vi "数字量输入配置.vi"() -> ()   [LabVIEW 2010]
panel:
  in  "数组":u16[](array[numeric]) format="%x"
  in  "保持输入":bool
  out "同步_A2":i32
  out "同步_A1":i32
  in  "数组_输入值":enum16{"0", "1"}[][](array[ring])
  in  "数组_选择?":bool[][](array[boolean])
  in  "btn_置1_5":bool
  in  "btn_置1_4":bool
  in  "btn_置1_3":bool
  in  "btn_置1_2":bool
  in  "btn_全选_5":bool
  in  "btn_全选_4":bool
  in  "btn_全选_3":bool
  in  "btn_全选_2":bool
  in  "btn_置1_1":bool
  in  "btn_全选_1":bool
  in  "CAN端口":u16
  out "light_80":bool
  out "light_79":bool
  out "light_78":bool
  out "light_77":bool
  out "light_76":bool
  out "light_75":bool
  out "light_74":bool
  out "light_73":bool
  out "light_72":bool
  out "light_71":bool
  out "light_70":bool
  out "light_69":bool
  out "light_68":bool
  out "light_67":bool
  out "light_66":bool
  out "light_65":bool
  in  "输入值_73":enum16{"0", "1"}(ring)
  in  "输入值_80":enum16{"0", "1"}(ring)
  in  "输入值_79":enum16{"0", "1"}(ring)
  in  "输入值_78":enum16{"0", "1"}(ring)
  in  "输入值_77":enum16{"0", "1"}(ring)
  in  "输入值_76":enum16{"0", "1"}(ring)
  in  "输入值_75":enum16{"0", "1"}(ring)
  in  "输入值_74":enum16{"0", "1"}(ring)
  in  "输入值_65":enum16{"0", "1"}(ring)
  in  "输入值_72":enum16{"0", "1"}(ring)
  in  "输入值_71":enum16{"0", "1"}(ring)
  in  "输入值_70":enum16{"0", "1"}(ring)
  in  "输入值_69":enum16{"0", "1"}(ring)
  in  "输入值_68":enum16{"0", "1"}(ring)
  in  "输入值_67":enum16{"0", "1"}(ring)
  in  "输入值_66":enum16{"0", "1"}(ring)
  in  "单选_第73路":bool
  in  "单选_第80路":bool
  in  "单选_第79路":bool
  in  "单选_第78路":bool
  in  "单选_第77路":bool
  in  "单选_第76路":bool
  in  "单选_第75路":bool
  in  "单选_第74路":bool
  in  "单选_第65路":bool
  in  "单选_第72路":bool
  in  "单选_第71路":bool
  in  "单选_第70路":bool
  in  "单选_第69路":bool
  in  "单选_第68路":bool
  in  "单选_第67路":bool
  in  "单选_第66路":bool
  out "light_64":bool
  out "light_63":bool
  out "light_62":bool
  out "light_61":bool
  out "light_60":bool
  out "light_59":bool
  out "light_58":bool
  out "light_57":bool
  out "light_56":bool
  out "light_55":bool
  out "light_54":bool
  out "light_53":bool
  out "light_52":bool
  out "light_51":bool
  out "light_50":bool
  out "light_49":bool
  in  "输入值_57":enum16{"0", "1"}(ring)
  in  "输入值_64":enum16{"0", "1"}(ring)
  in  "输入值_63":enum16{"0", "1"}(ring)
  in  "输入值_62":enum16{"0", "1"}(ring)
  in  "输入值_61":enum16{"0", "1"}(ring)
  in  "输入值_60":enum16{"0", "1"}(ring)
  in  "输入值_59":enum16{"0", "1"}(ring)
  in  "输入值_58":enum16{"0", "1"}(ring)
  in  "输入值_49":enum16{"0", "1"}(ring)
  in  "输入值_56":enum16{"0", "1"}(ring)
  in  "输入值_55":enum16{"0", "1"}(ring)
  in  "输入值_54":enum16{"0", "1"}(ring)
  in  "输入值_53":enum16{"0", "1"}(ring)
  in  "输入值_52":enum16{"0", "1"}(ring)
  in  "输入值_51":enum16{"0", "1"}(ring)
  in  "输入值_50":enum16{"0", "1"}(ring)
  in  "单选_第57路":bool
  in  "单选_第64路":bool
  in  "单选_第63路":bool
  in  "单选_第62路":bool
  in  "单选_第61路":bool
  in  "单选_第60路":bool
  in  "单选_第59路":bool
  in  "单选_第58路":bool
  in  "单选_第49路":bool
  in  "单选_第56路":bool
  in  "单选_第55路":bool
  in  "单选_第54路":bool
  in  "单选_第53路":bool
  in  "单选_第52路":bool
  in  "单选_第51路":bool
  in  "单选_第50路":bool
  out "light_48":bool
  out "light_47":bool
  out "light_46":bool
  out "light_45":bool
  out "light_44":bool
  out "light_43":bool
  out "light_42":bool
  out "light_41":bool
  out "light_40":bool
  out "light_39":bool
  out "light_38":bool
  out "light_37":bool
  out "light_36":bool
  out "light_35":bool
  out "light_34":bool
  out "light_33":bool
  in  "输入值_41":enum16{"0", "1"}(ring)
  in  "输入值_48":enum16{"0", "1"}(ring)
  in  "输入值_47":enum16{"0", "1"}(ring)
  in  "输入值_46":enum16{"0", "1"}(ring)
  in  "输入值_45":enum16{"0", "1"}(ring)
  in  "输入值_44":enum16{"0", "1"}(ring)
  in  "输入值_43":enum16{"0", "1"}(ring)
  in  "输入值_42":enum16{"0", "1"}(ring)
  in  "输入值_33":enum16{"0", "1"}(ring)
  in  "输入值_40":enum16{"0", "1"}(ring)
  in  "输入值_39":enum16{"0", "1"}(ring)
  in  "输入值_38":enum16{"0", "1"}(ring)
  in  "输入值_37":enum16{"0", "1"}(ring)
  in  "输入值_36":enum16{"0", "1"}(ring)
  in  "输入值_35":enum16{"0", "1"}(ring)
  in  "输入值_34":enum16{"0", "1"}(ring)
  in  "单选_第41路":bool
  in  "单选_第48路":bool
  in  "单选_第47路":bool
  in  "单选_第46路":bool
  in  "单选_第45路":bool
  in  "单选_第44路":bool
  in  "单选_第43路":bool
  in  "单选_第42路":bool
  in  "单选_第33路":bool
  in  "单选_第40路":bool
  in  "单选_第39路":bool
  in  "单选_第38路":bool
  in  "单选_第37路":bool
  in  "单选_第36路":bool
  in  "单选_第35路":bool
  in  "单选_第34路":bool
  out "light_32":bool
  out "light_31":bool
  out "light_30":bool
  out "light_29":bool
  out "light_28":bool
  out "light_27":bool
  out "light_26":bool
  out "light_25":bool
  out "light_24":bool
  out "light_23":bool
  out "light_22":bool
  out "light_21":bool
  out "light_20":bool
  out "light_19":bool
  out "light_18":bool
  out "light_17":bool
  in  "输入值_25":enum16{"0", "1"}(ring)
  in  "输入值_32":enum16{"0", "1"}(ring)
  in  "输入值_31":enum16{"0", "1"}(ring)
  in  "输入值_30":enum16{"0", "1"}(ring)
  in  "输入值_29":enum16{"0", "1"}(ring)
  in  "输入值_28":enum16{"0", "1"}(ring)
  in  "输入值_27":enum16{"0", "1"}(ring)
  in  "输入值_26":enum16{"0", "1"}(ring)
  in  "输入值_17":enum16{"0", "1"}(ring)
  in  "输入值_24":enum16{"0", "1"}(ring)
  in  "输入值_23":enum16{"0", "1"}(ring)
  in  "输入值_22":enum16{"0", "1"}(ring)
  in  "输入值_21":enum16{"0", "1"}(ring)
  in  "输入值_20":enum16{"0", "1"}(ring)
  in  "输入值_19":enum16{"0", "1"}(ring)
  in  "输入值_18":enum16{"0", "1"}(ring)
  in  "单选_第25路":bool
  in  "单选_第32路":bool
  in  "单选_第31路":bool
  in  "单选_第30路":bool
  in  "单选_第29路":bool
  in  "单选_第28路":bool
  in  "单选_第27路":bool
  in  "单选_第26路":bool
  in  "单选_第17路":bool
  in  "单选_第24路":bool
  in  "单选_第23路":bool
  in  "单选_第22路":bool
  in  "单选_第21路":bool
  in  "单选_第20路":bool
  in  "单选_第19路":bool
  in  "单选_第18路":bool
  in  "D_IN_5":string[][](table) caption="表格"
  in  "D_IN_4":string[][](table) caption="表格"
  in  "D_IN_3":string[][](table) caption="表格"
  in  "D_IN_2":string[][](table) caption="表格"
  out "light_16":bool
  out "light_15":bool
  out "light_14":bool
  out "light_13":bool
  out "light_12":bool
  out "light_11":bool
  out "light_10":bool
  out "light_9":bool
  out "light_8":bool
  out "light_7":bool
  out "light_6":bool
  out "light_5":bool
  out "light_4":bool
  out "light_3":bool
  out "light_2":bool
  out "light_1":bool
  in  "输入值_9":enum16{"0", "1"}(ring)
  in  "输入值_16":enum16{"0", "1"}(ring)
  in  "输入值_15":enum16{"0", "1"}(ring)
  in  "输入值_14":enum16{"0", "1"}(ring)
  in  "输入值_13":enum16{"0", "1"}(ring)
  in  "输入值_12":enum16{"0", "1"}(ring)
  in  "输入值_11":enum16{"0", "1"}(ring)
  in  "输入值_10":enum16{"0", "1"}(ring)
  in  "输入值_1":enum16{"0", "1"}(ring)
  in  "输入值_8":enum16{"0", "1"}(ring)
  in  "输入值_7":enum16{"0", "1"}(ring)
  in  "输入值_6":enum16{"0", "1"}(ring)
  in  "输入值_5":enum16{"0", "1"}(ring)
  in  "输入值_4":enum16{"0", "1"}(ring)
  in  "输入值_3":enum16{"0", "1"}(ring)
  in  "输入值_2":enum16{"0", "1"}(ring)
  in  "单选_第9路":bool
  in  "单选_第16路":bool
  in  "单选_第15路":bool
  in  "单选_第14路":bool
  in  "单选_第13路":bool
  in  "单选_第12路":bool
  in  "单选_第11路":bool
  in  "单选_第10路":bool
  in  "单选_第1路":bool
  in  "单选_第8路":bool
  in  "单选_第7路":bool
  in  "单选_第6路":bool
  in  "单选_第5路":bool
  in  "单选_第4路":bool
  in  "单选_第3路":bool
  in  "单选_第2路":bool
  in  "D_IN_1":string[][](table) caption="表格"
  out "关闭？":bool
  out "测试结论":string
  in  "btn_置0":bool
  in  "btn_置1":bool
  in  "btn_反选":bool
  in  "btn_全选":bool
  in  "btn_关闭":bool
  in  "btn_开始试验":bool
  # "第一组数字量输入"
  # "第二组数字量输入"
  # "第三组数字量输入"
  # "第四组数字量输入"
  # "第五组数字量输入(I/O)"
  # "测试结论："
  # "5X16"
  # "5X16"
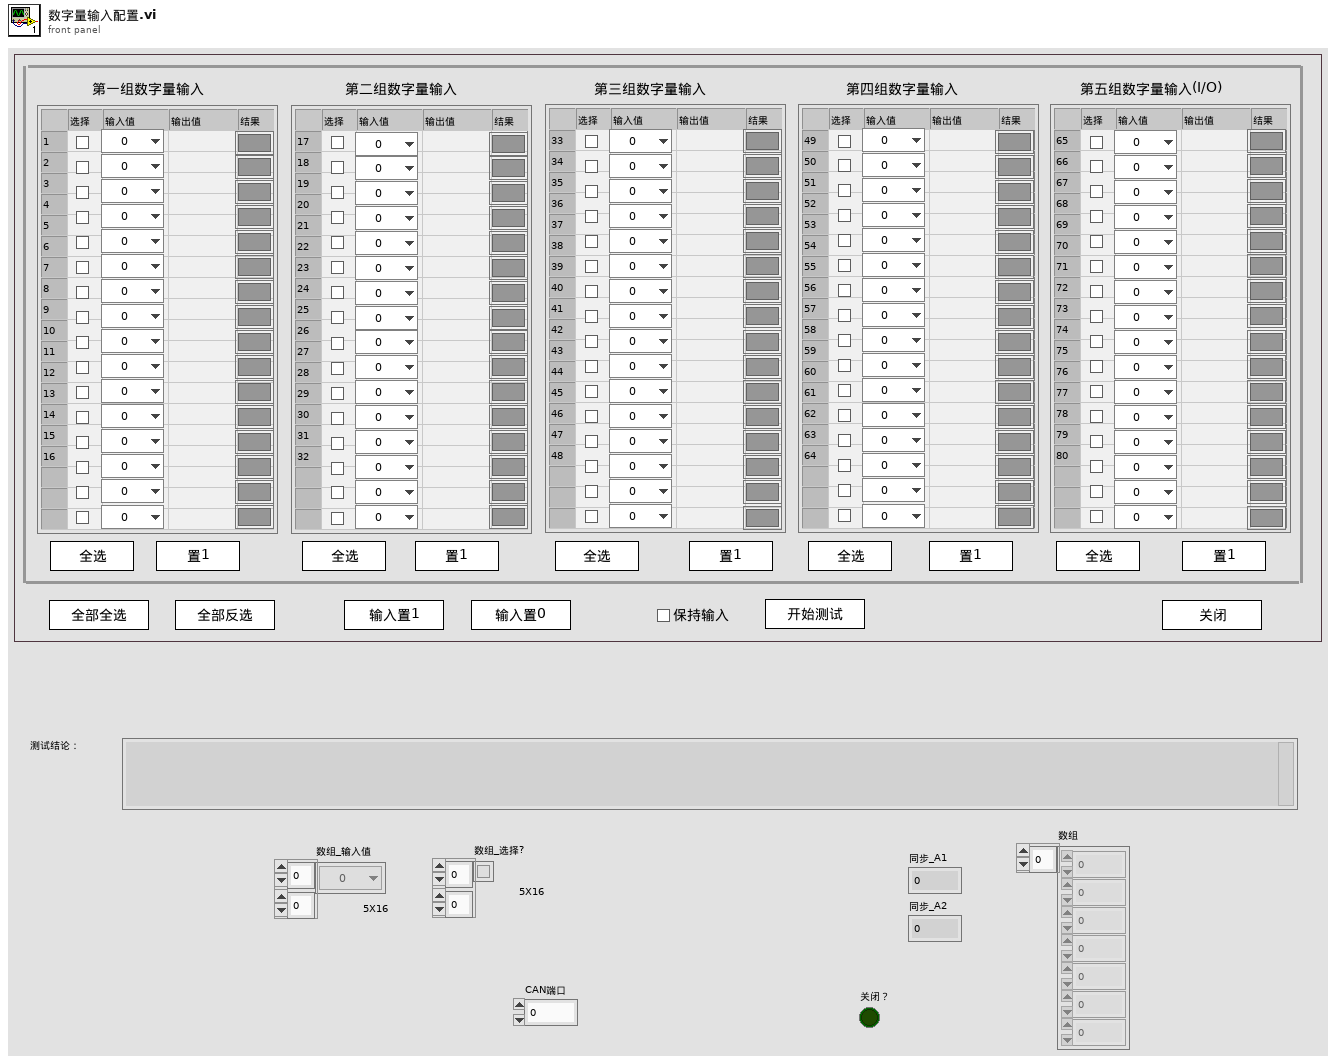
[diagram p1: front panel]
types:
  T1 = enum8{"Enabled", "Disabled", "Disabled and Grayed Out"}
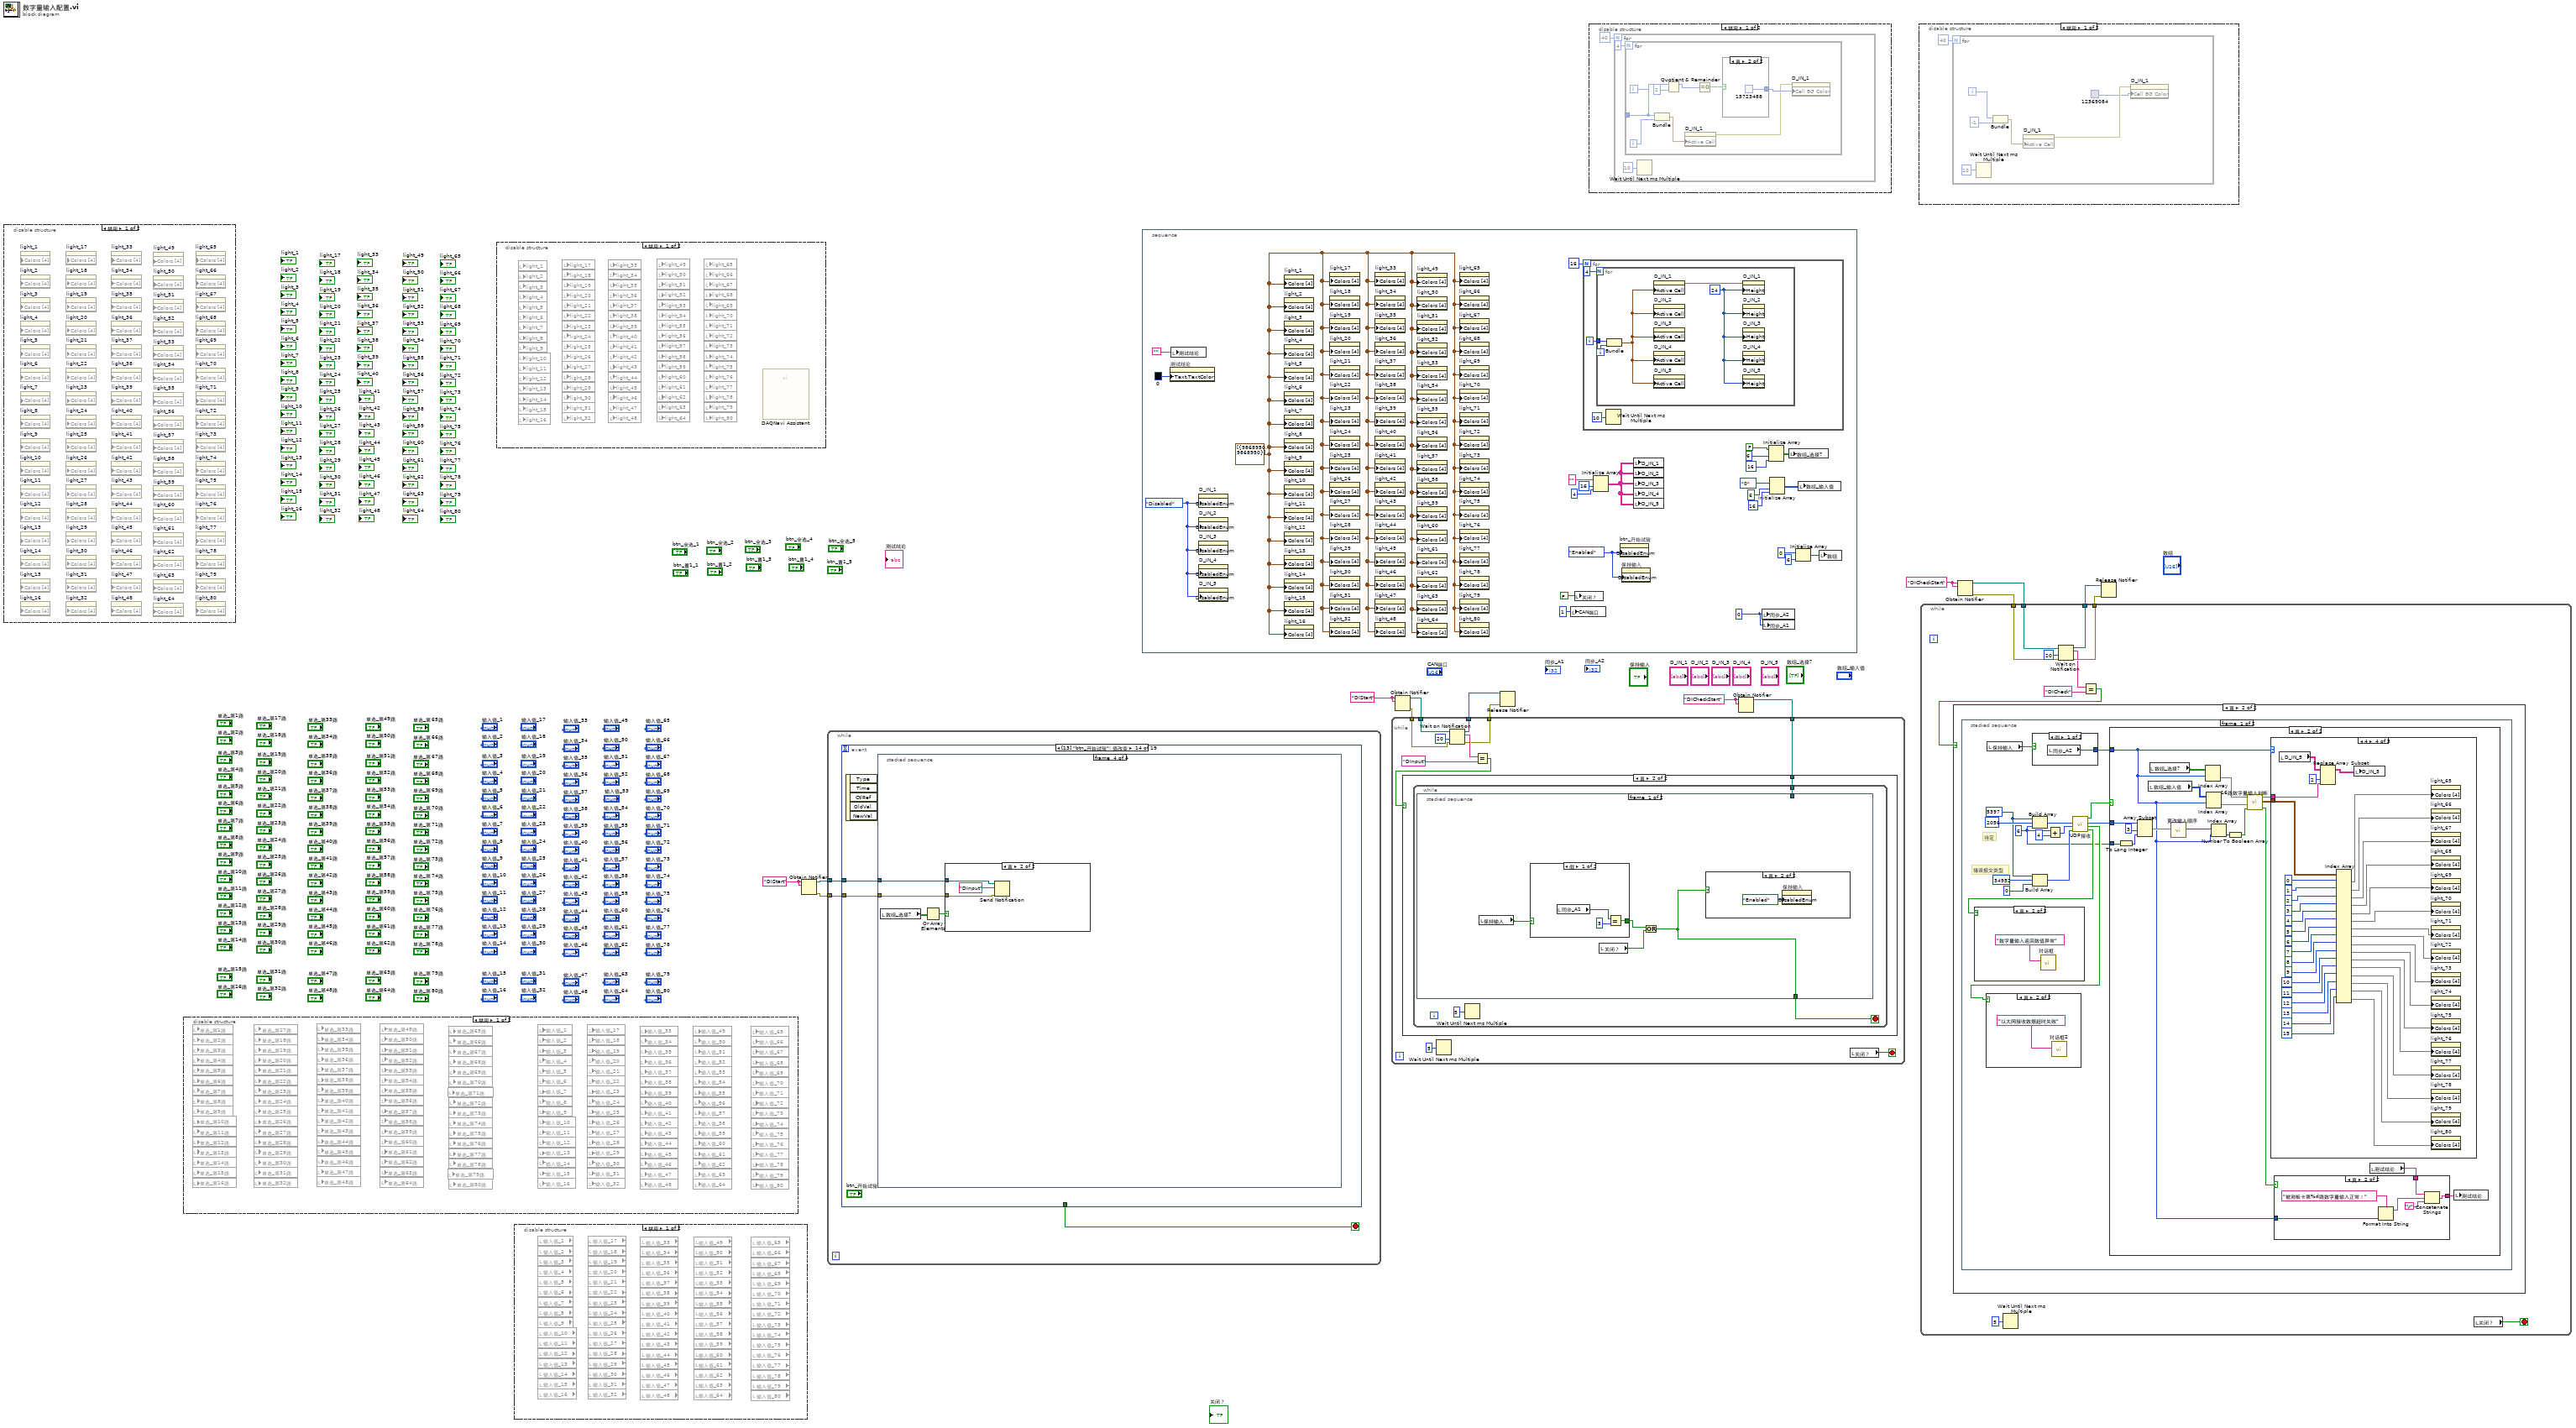
[diagram p0: block diagram]
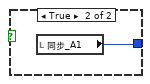
[diagram p3: hidden frame]
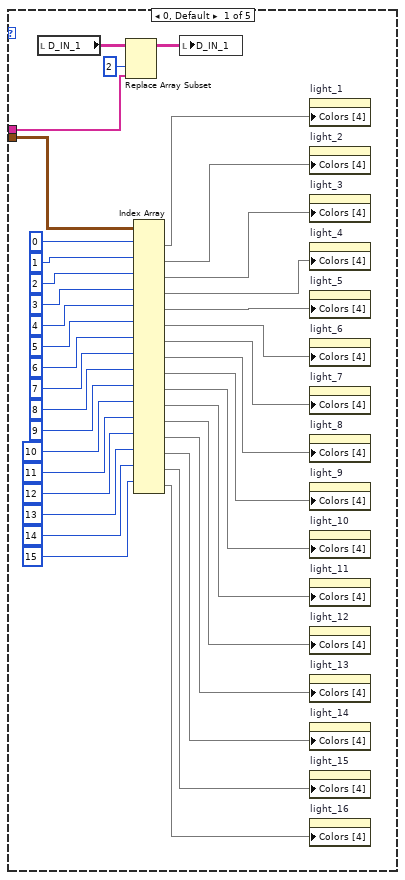
[diagram p7: hidden frame]
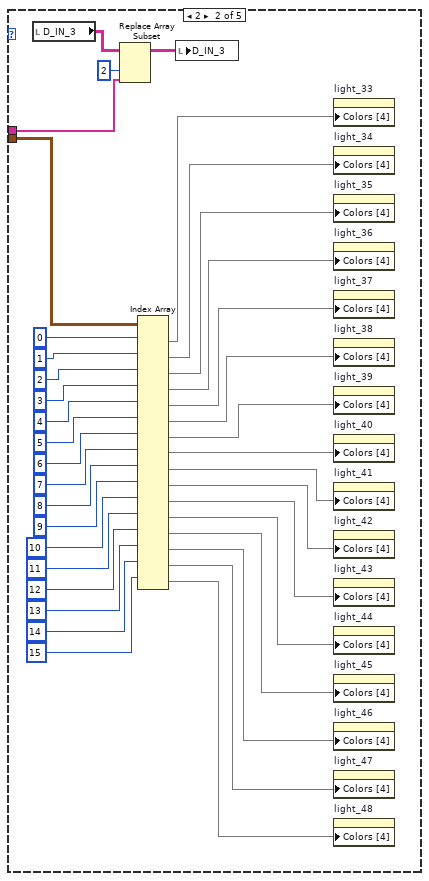
[diagram p8: hidden frame]
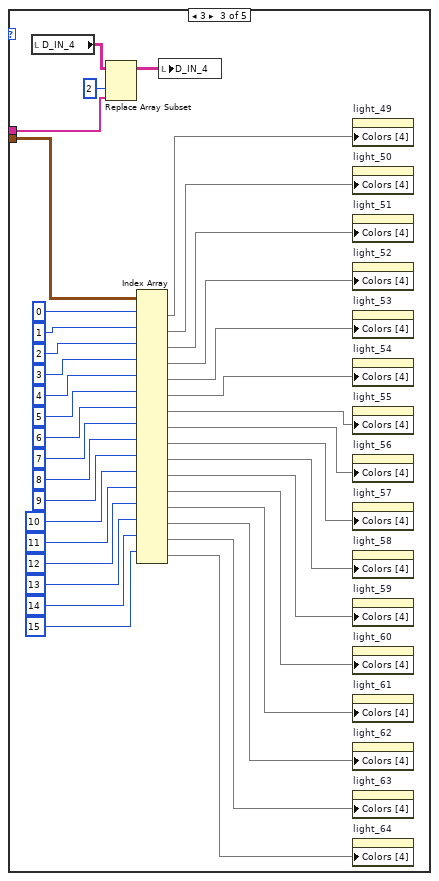
[diagram p9: hidden frame]
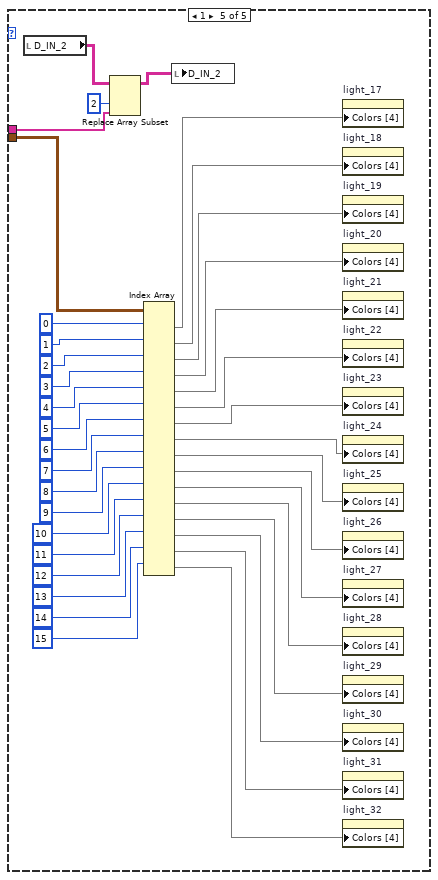
[diagram p10: hidden frame]
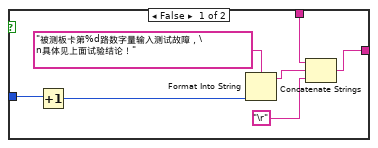
[diagram p11: hidden frame]
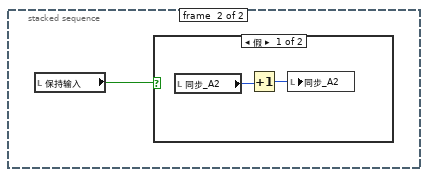
[diagram p12: hidden frame]
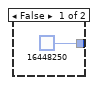
[diagram p15: hidden frame]
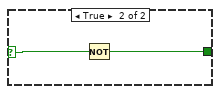
[diagram p19: hidden frame]
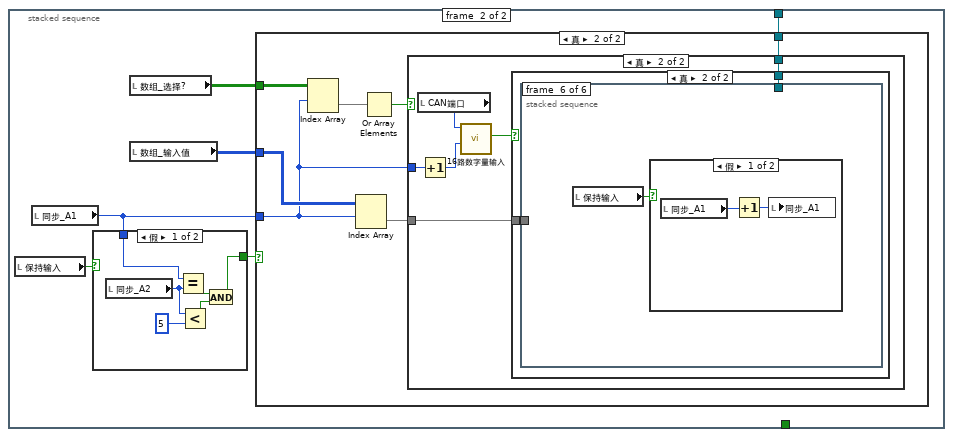
[diagram p20: hidden frame]
diagram:
  w2 = "DICheckStart" ("名称（未命名）")
  w5 = "DIStart" ("名称（未命名）")
  w10 = "DICheckStart" ("名称（未命名）")
  w11 = "DIStart" ("名称（未命名）")
  n1 = disable-structure shown="禁用" {
    frame Disabled {
      n2 = property on="light_1" class="Bool (严格)" props=["Colors [4]"]() -> ()  [unwired: 3 in, 2 out]
      n3 = property on="light_2" class="Bool (严格)" props=["Colors [4]"]() -> ()  [unwired: 3 in, 2 out]
      n4 = property on="light_3" class="Bool (严格)" props=["Colors [4]"]() -> ()  [unwired: 3 in, 2 out]
      n5 = property on="light_4" class="Bool (严格)" props=["Colors [4]"]() -> ()  [unwired: 3 in, 2 out]
      n6 = property on="light_5" class="Bool (严格)" props=["Colors [4]"]() -> ()  [unwired: 3 in, 2 out]
      n7 = property on="light_6" class="Bool (严格)" props=["Colors [4]"]() -> ()  [unwired: 3 in, 2 out]
      n8 = property on="light_7" class="Bool (严格)" props=["Colors [4]"]() -> ()  [unwired: 3 in, 2 out]
      n9 = property on="light_8" class="Bool (严格)" props=["Colors [4]"]() -> ()  [unwired: 3 in, 2 out]
      n10 = property on="light_9" class="Bool (严格)" props=["Colors [4]"]() -> ()  [unwired: 3 in, 2 out]
      n11 = property on="light_10" class="Bool (严格)" props=["Colors [4]"]() -> ()  [unwired: 3 in, 2 out]
      n12 = property on="light_11" class="Bool (严格)" props=["Colors [4]"]() -> ()  [unwired: 3 in, 2 out]
      n13 = property on="light_12" class="Bool (严格)" props=["Colors [4]"]() -> ()  [unwired: 3 in, 2 out]
      n14 = property on="light_13" class="Bool (严格)" props=["Colors [4]"]() -> ()  [unwired: 3 in, 2 out]
      n15 = property on="light_14" class="Bool (严格)" props=["Colors [4]"]() -> ()  [unwired: 3 in, 2 out]
      n16 = property on="light_15" class="Bool (严格)" props=["Colors [4]"]() -> ()  [unwired: 3 in, 2 out]
      n17 = property on="light_16" class="Bool (严格)" props=["Colors [4]"]() -> ()  [unwired: 3 in, 2 out]
      n18 = property on="light_17" class="Bool (严格)" props=["Colors [4]"]() -> ()  [unwired: 3 in, 2 out]
      n19 = property on="light_18" class="Bool (严格)" props=["Colors [4]"]() -> ()  [unwired: 3 in, 2 out]
      n20 = property on="light_19" class="Bool (严格)" props=["Colors [4]"]() -> ()  [unwired: 3 in, 2 out]
      n21 = property on="light_20" class="Bool (严格)" props=["Colors [4]"]() -> ()  [unwired: 3 in, 2 out]
      n22 = property on="light_21" class="Bool (严格)" props=["Colors [4]"]() -> ()  [unwired: 3 in, 2 out]
      n23 = property on="light_22" class="Bool (严格)" props=["Colors [4]"]() -> ()  [unwired: 3 in, 2 out]
      n24 = property on="light_23" class="Bool (严格)" props=["Colors [4]"]() -> ()  [unwired: 3 in, 2 out]
      n25 = property on="light_24" class="Bool (严格)" props=["Colors [4]"]() -> ()  [unwired: 3 in, 2 out]
      n26 = property on="light_25" class="Bool (严格)" props=["Colors [4]"]() -> ()  [unwired: 3 in, 2 out]
      n27 = property on="light_26" class="Bool (严格)" props=["Colors [4]"]() -> ()  [unwired: 3 in, 2 out]
      n28 = property on="light_27" class="Bool (严格)" props=["Colors [4]"]() -> ()  [unwired: 3 in, 2 out]
      n29 = property on="light_28" class="Bool (严格)" props=["Colors [4]"]() -> ()  [unwired: 3 in, 2 out]
      n30 = property on="light_29" class="Bool (严格)" props=["Colors [4]"]() -> ()  [unwired: 3 in, 2 out]
      n31 = property on="light_30" class="Bool (严格)" props=["Colors [4]"]() -> ()  [unwired: 3 in, 2 out]
      n32 = property on="light_31" class="Bool (严格)" props=["Colors [4]"]() -> ()  [unwired: 3 in, 2 out]
      n33 = property on="light_32" class="Bool (严格)" props=["Colors [4]"]() -> ()  [unwired: 3 in, 2 out]
      n34 = property on="light_33" class="Bool (严格)" props=["Colors [4]"]() -> ()  [unwired: 3 in, 2 out]
      n35 = property on="light_34" class="Bool (严格)" props=["Colors [4]"]() -> ()  [unwired: 3 in, 2 out]
      n36 = property on="light_35" class="Bool (严格)" props=["Colors [4]"]() -> ()  [unwired: 3 in, 2 out]
      n37 = property on="light_36" class="Bool (严格)" props=["Colors [4]"]() -> ()  [unwired: 3 in, 2 out]
      n38 = property on="light_37" class="Bool (严格)" props=["Colors [4]"]() -> ()  [unwired: 3 in, 2 out]
      n39 = property on="light_38" class="Bool (严格)" props=["Colors [4]"]() -> ()  [unwired: 3 in, 2 out]
      n40 = property on="light_39" class="Bool (严格)" props=["Colors [4]"]() -> ()  [unwired: 3 in, 2 out]
      n41 = property on="light_40" class="Bool (严格)" props=["Colors [4]"]() -> ()  [unwired: 3 in, 2 out]
      n42 = property on="light_41" class="Bool (严格)" props=["Colors [4]"]() -> ()  [unwired: 3 in, 2 out]
      n43 = property on="light_42" class="Bool (严格)" props=["Colors [4]"]() -> ()  [unwired: 3 in, 2 out]
      n44 = property on="light_43" class="Bool (严格)" props=["Colors [4]"]() -> ()  [unwired: 3 in, 2 out]
      n45 = property on="light_44" class="Bool (严格)" props=["Colors [4]"]() -> ()  [unwired: 3 in, 2 out]
      n46 = property on="light_45" class="Bool (严格)" props=["Colors [4]"]() -> ()  [unwired: 3 in, 2 out]
      n47 = property on="light_46" class="Bool (严格)" props=["Colors [4]"]() -> ()  [unwired: 3 in, 2 out]
      n48 = property on="light_47" class="Bool (严格)" props=["Colors [4]"]() -> ()  [unwired: 3 in, 2 out]
      n49 = property on="light_48" class="Bool (严格)" props=["Colors [4]"]() -> ()  [unwired: 3 in, 2 out]
      n50 = property on="light_49" class="Bool (严格)" props=["Colors [4]"]() -> ()  [unwired: 3 in, 2 out]
      n51 = property on="light_50" class="Bool (严格)" props=["Colors [4]"]() -> ()  [unwired: 3 in, 2 out]
      n52 = property on="light_51" class="Bool (严格)" props=["Colors [4]"]() -> ()  [unwired: 3 in, 2 out]
      n53 = property on="light_52" class="Bool (严格)" props=["Colors [4]"]() -> ()  [unwired: 3 in, 2 out]
      n54 = property on="light_53" class="Bool (严格)" props=["Colors [4]"]() -> ()  [unwired: 3 in, 2 out]
      n55 = property on="light_54" class="Bool (严格)" props=["Colors [4]"]() -> ()  [unwired: 3 in, 2 out]
      n56 = property on="light_55" class="Bool (严格)" props=["Colors [4]"]() -> ()  [unwired: 3 in, 2 out]
      n57 = property on="light_56" class="Bool (严格)" props=["Colors [4]"]() -> ()  [unwired: 3 in, 2 out]
      n58 = property on="light_57" class="Bool (严格)" props=["Colors [4]"]() -> ()  [unwired: 3 in, 2 out]
      n59 = property on="light_58" class="Bool (严格)" props=["Colors [4]"]() -> ()  [unwired: 3 in, 2 out]
      n60 = property on="light_59" class="Bool (严格)" props=["Colors [4]"]() -> ()  [unwired: 3 in, 2 out]
      n61 = property on="light_60" class="Bool (严格)" props=["Colors [4]"]() -> ()  [unwired: 3 in, 2 out]
      n62 = property on="light_61" class="Bool (严格)" props=["Colors [4]"]() -> ()  [unwired: 3 in, 2 out]
      n63 = property on="light_62" class="Bool (严格)" props=["Colors [4]"]() -> ()  [unwired: 3 in, 2 out]
      n64 = property on="light_63" class="Bool (严格)" props=["Colors [4]"]() -> ()  [unwired: 3 in, 2 out]
      n65 = property on="light_64" class="Bool (严格)" props=["Colors [4]"]() -> ()  [unwired: 3 in, 2 out]
      n66 = property on="light_65" class="Bool (严格)" props=["Colors [4]"]() -> ()  [unwired: 3 in, 2 out]
      n67 = property on="light_66" class="Bool (严格)" props=["Colors [4]"]() -> ()  [unwired: 3 in, 2 out]
      n68 = property on="light_67" class="Bool (严格)" props=["Colors [4]"]() -> ()  [unwired: 3 in, 2 out]
      n69 = property on="light_68" class="Bool (严格)" props=["Colors [4]"]() -> ()  [unwired: 3 in, 2 out]
      n70 = property on="light_69" class="Bool (严格)" props=["Colors [4]"]() -> ()  [unwired: 3 in, 2 out]
      n71 = property on="light_70" class="Bool (严格)" props=["Colors [4]"]() -> ()  [unwired: 3 in, 2 out]
      n72 = property on="light_71" class="Bool (严格)" props=["Colors [4]"]() -> ()  [unwired: 3 in, 2 out]
      n73 = property on="light_72" class="Bool (严格)" props=["Colors [4]"]() -> ()  [unwired: 3 in, 2 out]
      n74 = property on="light_73" class="Bool (严格)" props=["Colors [4]"]() -> ()  [unwired: 3 in, 2 out]
      n75 = property on="light_74" class="Bool (严格)" props=["Colors [4]"]() -> ()  [unwired: 3 in, 2 out]
      n76 = property on="light_75" class="Bool (严格)" props=["Colors [4]"]() -> ()  [unwired: 3 in, 2 out]
      n77 = property on="light_76" class="Bool (严格)" props=["Colors [4]"]() -> ()  [unwired: 3 in, 2 out]
      n78 = property on="light_77" class="Bool (严格)" props=["Colors [4]"]() -> ()  [unwired: 3 in, 2 out]
      n79 = property on="light_78" class="Bool (严格)" props=["Colors [4]"]() -> ()  [unwired: 3 in, 2 out]
      n80 = property on="light_79" class="Bool (严格)" props=["Colors [4]"]() -> ()  [unwired: 3 in, 2 out]
      n81 = property on="light_80" class="Bool (严格)" props=["Colors [4]"]() -> ()  [unwired: 3 in, 2 out]
    }
    frame Enabled {
    }
  }
  n82 = disable-structure shown="禁用" {
    frame Disabled {
      n83 = local read "单选_第1路"() -> ()  [unwired: 1 in]
      n84 = local read "单选_第2路"() -> ()  [unwired: 1 in]
      n85 = local read "单选_第3路"() -> ()  [unwired: 1 in]
      n86 = local read "单选_第4路"() -> ()  [unwired: 1 in]
      n87 = local read "单选_第5路"() -> ()  [unwired: 1 in]
      n88 = local read "单选_第6路"() -> ()  [unwired: 1 in]
      n89 = local read "单选_第7路"() -> ()  [unwired: 1 in]
      n90 = local read "单选_第8路"() -> ()  [unwired: 1 in]
      n91 = local read "单选_第9路"() -> ()  [unwired: 1 in]
      n92 = local read "单选_第10路"() -> ()  [unwired: 1 in]
      n93 = local read "单选_第11路"() -> ()  [unwired: 1 in]
      n94 = local read "单选_第12路"() -> ()  [unwired: 1 in]
      n95 = local read "单选_第13路"() -> ()  [unwired: 1 in]
      n96 = local read "单选_第14路"() -> ()  [unwired: 1 in]
      n97 = local read "单选_第15路"() -> ()  [unwired: 1 in]
      n98 = local read "单选_第16路"() -> ()  [unwired: 1 in]
      n99 = local read "单选_第17路"() -> ()  [unwired: 1 in]
      n100 = local read "单选_第18路"() -> ()  [unwired: 1 in]
      n101 = local read "单选_第19路"() -> ()  [unwired: 1 in]
      n102 = local read "单选_第20路"() -> ()  [unwired: 1 in]
      n103 = local read "单选_第21路"() -> ()  [unwired: 1 in]
      n104 = local read "单选_第22路"() -> ()  [unwired: 1 in]
      n105 = local read "单选_第23路"() -> ()  [unwired: 1 in]
      n106 = local read "单选_第24路"() -> ()  [unwired: 1 in]
      n107 = local read "单选_第25路"() -> ()  [unwired: 1 in]
      n108 = local read "单选_第26路"() -> ()  [unwired: 1 in]
      n109 = local read "单选_第27路"() -> ()  [unwired: 1 in]
      n110 = local read "单选_第28路"() -> ()  [unwired: 1 in]
      n111 = local read "单选_第29路"() -> ()  [unwired: 1 in]
      n112 = local read "单选_第30路"() -> ()  [unwired: 1 in]
      n113 = local read "单选_第31路"() -> ()  [unwired: 1 in]
      n114 = local read "单选_第32路"() -> ()  [unwired: 1 in]
      n115 = local read "单选_第33路"() -> ()  [unwired: 1 in]
      n116 = local read "单选_第34路"() -> ()  [unwired: 1 in]
      n117 = local read "单选_第35路"() -> ()  [unwired: 1 in]
      n118 = local read "单选_第36路"() -> ()  [unwired: 1 in]
      n119 = local read "单选_第37路"() -> ()  [unwired: 1 in]
      n120 = local read "单选_第38路"() -> ()  [unwired: 1 in]
      n121 = local read "单选_第39路"() -> ()  [unwired: 1 in]
      n122 = local read "单选_第40路"() -> ()  [unwired: 1 in]
      n123 = local read "单选_第41路"() -> ()  [unwired: 1 in]
      n124 = local read "单选_第42路"() -> ()  [unwired: 1 in]
      n125 = local read "单选_第43路"() -> ()  [unwired: 1 in]
      n126 = local read "单选_第44路"() -> ()  [unwired: 1 in]
      n127 = local read "单选_第45路"() -> ()  [unwired: 1 in]
      n128 = local read "单选_第46路"() -> ()  [unwired: 1 in]
      n129 = local read "单选_第47路"() -> ()  [unwired: 1 in]
      n130 = local read "单选_第48路"() -> ()  [unwired: 1 in]
      n131 = local read "单选_第49路"() -> ()  [unwired: 1 in]
      n132 = local read "单选_第50路"() -> ()  [unwired: 1 in]
      n133 = local read "单选_第51路"() -> ()  [unwired: 1 in]
      n134 = local read "单选_第52路"() -> ()  [unwired: 1 in]
      n135 = local read "单选_第53路"() -> ()  [unwired: 1 in]
      n136 = local read "单选_第54路"() -> ()  [unwired: 1 in]
      n137 = local read "单选_第55路"() -> ()  [unwired: 1 in]
      n138 = local read "单选_第56路"() -> ()  [unwired: 1 in]
      n139 = local read "单选_第57路"() -> ()  [unwired: 1 in]
      n140 = local read "单选_第58路"() -> ()  [unwired: 1 in]
      n141 = local read "单选_第59路"() -> ()  [unwired: 1 in]
      n142 = local read "单选_第60路"() -> ()  [unwired: 1 in]
      n143 = local read "单选_第61路"() -> ()  [unwired: 1 in]
      n144 = local read "单选_第62路"() -> ()  [unwired: 1 in]
      n145 = local read "单选_第63路"() -> ()  [unwired: 1 in]
      n146 = local read "单选_第64路"() -> ()  [unwired: 1 in]
      n147 = local read "单选_第71路"() -> ()  [unwired: 1 in]
      n148 = local read "单选_第79路"() -> ()  [unwired: 1 in]
      n149 = local read "单选_第65路"() -> ()  [unwired: 1 in]
      n150 = local read "单选_第66路"() -> ()  [unwired: 1 in]
      n151 = local read "单选_第67路"() -> ()  [unwired: 1 in]
      n152 = local read "单选_第68路"() -> ()  [unwired: 1 in]
      n153 = local read "单选_第69路"() -> ()  [unwired: 1 in]
      n154 = local read "单选_第70路"() -> ()  [unwired: 1 in]
      n155 = local read "单选_第72路"() -> ()  [unwired: 1 in]
      n156 = local read "单选_第73路"() -> ()  [unwired: 1 in]
      n157 = local read "单选_第74路"() -> ()  [unwired: 1 in]
      n158 = local read "单选_第75路"() -> ()  [unwired: 1 in]
      n159 = local read "单选_第76路"() -> ()  [unwired: 1 in]
      n160 = local read "单选_第77路"() -> ()  [unwired: 1 in]
      n161 = local read "单选_第78路"() -> ()  [unwired: 1 in]
      n162 = local read "单选_第80路"() -> ()  [unwired: 1 in]
      n163 = local read "输入值_1"() -> ()  [unwired: 1 in]
      n164 = local read "输入值_2"() -> ()  [unwired: 1 in]
      n165 = local read "输入值_3"() -> ()  [unwired: 1 in]
      n166 = local read "输入值_4"() -> ()  [unwired: 1 in]
      n167 = local read "输入值_5"() -> ()  [unwired: 1 in]
      n168 = local read "输入值_6"() -> ()  [unwired: 1 in]
      n169 = local read "输入值_7"() -> ()  [unwired: 1 in]
      n170 = local read "输入值_8"() -> ()  [unwired: 1 in]
      n171 = local read "输入值_9"() -> ()  [unwired: 1 in]
      n172 = local read "输入值_10"() -> ()  [unwired: 1 in]
      n173 = local read "输入值_11"() -> ()  [unwired: 1 in]
      n174 = local read "输入值_12"() -> ()  [unwired: 1 in]
      n175 = local read "输入值_13"() -> ()  [unwired: 1 in]
      n176 = local read "输入值_14"() -> ()  [unwired: 1 in]
      n177 = local read "输入值_15"() -> ()  [unwired: 1 in]
      n178 = local read "输入值_16"() -> ()  [unwired: 1 in]
      n179 = local read "输入值_17"() -> ()  [unwired: 1 in]
      n180 = local read "输入值_18"() -> ()  [unwired: 1 in]
      n181 = local read "输入值_19"() -> ()  [unwired: 1 in]
      n182 = local read "输入值_20"() -> ()  [unwired: 1 in]
      n183 = local read "输入值_21"() -> ()  [unwired: 1 in]
      n184 = local read "输入值_22"() -> ()  [unwired: 1 in]
      n185 = local read "输入值_23"() -> ()  [unwired: 1 in]
      n186 = local read "输入值_24"() -> ()  [unwired: 1 in]
      n187 = local read "输入值_25"() -> ()  [unwired: 1 in]
      n188 = local read "输入值_26"() -> ()  [unwired: 1 in]
      n189 = local read "输入值_27"() -> ()  [unwired: 1 in]
      n190 = local read "输入值_28"() -> ()  [unwired: 1 in]
      n191 = local read "输入值_29"() -> ()  [unwired: 1 in]
      n192 = local read "输入值_30"() -> ()  [unwired: 1 in]
      n193 = local read "输入值_31"() -> ()  [unwired: 1 in]
      n194 = local read "输入值_32"() -> ()  [unwired: 1 in]
      n195 = local read "输入值_33"() -> ()  [unwired: 1 in]
      n196 = local read "输入值_34"() -> ()  [unwired: 1 in]
      n197 = local read "输入值_35"() -> ()  [unwired: 1 in]
      n198 = local read "输入值_36"() -> ()  [unwired: 1 in]
      n199 = local read "输入值_37"() -> ()  [unwired: 1 in]
      n200 = local read "输入值_38"() -> ()  [unwired: 1 in]
      n201 = local read "输入值_39"() -> ()  [unwired: 1 in]
      n202 = local read "输入值_40"() -> ()  [unwired: 1 in]
      n203 = local read "输入值_41"() -> ()  [unwired: 1 in]
      n204 = local read "输入值_42"() -> ()  [unwired: 1 in]
      n205 = local read "输入值_43"() -> ()  [unwired: 1 in]
      n206 = local read "输入值_44"() -> ()  [unwired: 1 in]
      n207 = local read "输入值_45"() -> ()  [unwired: 1 in]
      n208 = local read "输入值_46"() -> ()  [unwired: 1 in]
      n209 = local read "输入值_47"() -> ()  [unwired: 1 in]
      n210 = local read "输入值_48"() -> ()  [unwired: 1 in]
      n211 = local read "输入值_49"() -> ()  [unwired: 1 in]
      n212 = local read "输入值_50"() -> ()  [unwired: 1 in]
      n213 = local read "输入值_51"() -> ()  [unwired: 1 in]
      n214 = local read "输入值_52"() -> ()  [unwired: 1 in]
      n215 = local read "输入值_53"() -> ()  [unwired: 1 in]
      n216 = local read "输入值_54"() -> ()  [unwired: 1 in]
      n217 = local read "输入值_55"() -> ()  [unwired: 1 in]
      n218 = local read "输入值_56"() -> ()  [unwired: 1 in]
      n219 = local read "输入值_57"() -> ()  [unwired: 1 in]
      n220 = local read "输入值_58"() -> ()  [unwired: 1 in]
      n221 = local read "输入值_59"() -> ()  [unwired: 1 in]
      n222 = local read "输入值_60"() -> ()  [unwired: 1 in]
      n223 = local read "输入值_61"() -> ()  [unwired: 1 in]
      n224 = local read "输入值_62"() -> ()  [unwired: 1 in]
      n225 = local read "输入值_63"() -> ()  [unwired: 1 in]
      n226 = local read "输入值_64"() -> ()  [unwired: 1 in]
      n227 = local read "输入值_65"() -> ()  [unwired: 1 in]
      n228 = local read "输入值_66"() -> ()  [unwired: 1 in]
      n229 = local read "输入值_67"() -> ()  [unwired: 1 in]
      n230 = local read "输入值_68"() -> ()  [unwired: 1 in]
      n231 = local read "输入值_69"() -> ()  [unwired: 1 in]
      n232 = local read "输入值_70"() -> ()  [unwired: 1 in]
      n233 = local read "输入值_71"() -> ()  [unwired: 1 in]
      n234 = local read "输入值_72"() -> ()  [unwired: 1 in]
      n235 = local read "输入值_73"() -> ()  [unwired: 1 in]
      n236 = local read "输入值_74"() -> ()  [unwired: 1 in]
      n237 = local read "输入值_75"() -> ()  [unwired: 1 in]
      n238 = local read "输入值_76"() -> ()  [unwired: 1 in]
      n239 = local read "输入值_77"() -> ()  [unwired: 1 in]
      n240 = local read "输入值_78"() -> ()  [unwired: 1 in]
      n241 = local read "输入值_79"() -> ()  [unwired: 1 in]
      n242 = local read "输入值_80"() -> ()  [unwired: 1 in]
    }
    frame Enabled {
    }
  }
  n243 = disable-structure shown="禁用" {
    frame Disabled {
      n244 = local read "light_1"() -> ()  [unwired: 1 in]
      n245 = local read "light_2"() -> ()  [unwired: 1 in]
      n246 = local read "light_3"() -> ()  [unwired: 1 in]
      n247 = local read "light_4"() -> ()  [unwired: 1 in]
      n248 = local read "light_5"() -> ()  [unwired: 1 in]
      n249 = local read "light_6"() -> ()  [unwired: 1 in]
      n250 = local read "light_7"() -> ()  [unwired: 1 in]
      n251 = local read "light_8"() -> ()  [unwired: 1 in]
      n252 = local read "light_9"() -> ()  [unwired: 1 in]
      n253 = local read "light_10"() -> ()  [unwired: 1 in]
      n254 = local read "light_11"() -> ()  [unwired: 1 in]
      n255 = local read "light_12"() -> ()  [unwired: 1 in]
      n256 = local read "light_13"() -> ()  [unwired: 1 in]
      n257 = local read "light_14"() -> ()  [unwired: 1 in]
      n258 = local read "light_15"() -> ()  [unwired: 1 in]
      n259 = local read "light_16"() -> ()  [unwired: 1 in]
      n260 = local read "light_17"() -> ()  [unwired: 1 in]
      n261 = local read "light_18"() -> ()  [unwired: 1 in]
      n262 = local read "light_19"() -> ()  [unwired: 1 in]
      n263 = local read "light_20"() -> ()  [unwired: 1 in]
      n264 = local read "light_21"() -> ()  [unwired: 1 in]
      n265 = local read "light_22"() -> ()  [unwired: 1 in]
      n266 = local read "light_23"() -> ()  [unwired: 1 in]
      n267 = local read "light_24"() -> ()  [unwired: 1 in]
      n268 = local read "light_25"() -> ()  [unwired: 1 in]
      n269 = local read "light_26"() -> ()  [unwired: 1 in]
      n270 = local read "light_27"() -> ()  [unwired: 1 in]
      n271 = local read "light_28"() -> ()  [unwired: 1 in]
      n272 = local read "light_29"() -> ()  [unwired: 1 in]
      n273 = local read "light_30"() -> ()  [unwired: 1 in]
      n274 = local read "light_31"() -> ()  [unwired: 1 in]
      n275 = local read "light_32"() -> ()  [unwired: 1 in]
      n276 = local read "light_33"() -> ()  [unwired: 1 in]
      n277 = local read "light_34"() -> ()  [unwired: 1 in]
      n278 = local read "light_35"() -> ()  [unwired: 1 in]
      n279 = local read "light_36"() -> ()  [unwired: 1 in]
      n280 = local read "light_37"() -> ()  [unwired: 1 in]
      n281 = local read "light_38"() -> ()  [unwired: 1 in]
      n282 = local read "light_39"() -> ()  [unwired: 1 in]
      n283 = local read "light_40"() -> ()  [unwired: 1 in]
      n284 = local read "light_41"() -> ()  [unwired: 1 in]
      n285 = local read "light_42"() -> ()  [unwired: 1 in]
      n286 = local read "light_43"() -> ()  [unwired: 1 in]
      n287 = local read "light_44"() -> ()  [unwired: 1 in]
      n288 = local read "light_45"() -> ()  [unwired: 1 in]
      n289 = local read "light_46"() -> ()  [unwired: 1 in]
      n290 = local read "light_47"() -> ()  [unwired: 1 in]
      n291 = local read "light_48"() -> ()  [unwired: 1 in]
      n292 = local read "light_49"() -> ()  [unwired: 1 in]
      n293 = local read "light_50"() -> ()  [unwired: 1 in]
      n294 = local read "light_51"() -> ()  [unwired: 1 in]
      n295 = local read "light_52"() -> ()  [unwired: 1 in]
      n296 = local read "light_53"() -> ()  [unwired: 1 in]
      n297 = local read "light_54"() -> ()  [unwired: 1 in]
      n298 = local read "light_55"() -> ()  [unwired: 1 in]
      n299 = local read "light_56"() -> ()  [unwired: 1 in]
      n300 = local read "light_57"() -> ()  [unwired: 1 in]
      n301 = local read "light_58"() -> ()  [unwired: 1 in]
      n302 = local read "light_59"() -> ()  [unwired: 1 in]
      n303 = local read "light_60"() -> ()  [unwired: 1 in]
      n304 = local read "light_61"() -> ()  [unwired: 1 in]
      n305 = local read "light_62"() -> ()  [unwired: 1 in]
      n306 = local read "light_63"() -> ()  [unwired: 1 in]
      n307 = local read "light_64"() -> ()  [unwired: 1 in]
      n308 = local read "light_65"() -> ()  [unwired: 1 in]
      n309 = local read "light_66"() -> ()  [unwired: 1 in]
      n310 = local read "light_67"() -> ()  [unwired: 1 in]
      n311 = local read "light_68"() -> ()  [unwired: 1 in]
      n312 = local read "light_69"() -> ()  [unwired: 1 in]
      n313 = local read "light_70"() -> ()  [unwired: 1 in]
      n314 = local read "light_71"() -> ()  [unwired: 1 in]
      n315 = local read "light_72"() -> ()  [unwired: 1 in]
      n316 = local read "light_73"() -> ()  [unwired: 1 in]
      n317 = local read "light_74"() -> ()  [unwired: 1 in]
      n318 = local read "light_75"() -> ()  [unwired: 1 in]
      n319 = local read "light_76"() -> ()  [unwired: 1 in]
      n320 = local read "light_77"() -> ()  [unwired: 1 in]
      n321 = local read "light_78"() -> ()  [unwired: 1 in]
      n322 = local read "light_79"() -> ()  [unwired: 1 in]
      n323 = local read "light_80"() -> ()  [unwired: 1 in]
      n324 = call "DAQNavi Assistant"() -> ()  [unwired: 2 in, 18 out]
    }
    frame Enabled {
    }
  }
  n325 = disable-structure shown="禁用" {
    frame Disabled {
      n326 = local read "输入值_1"() -> ()  [unwired: 1 out]
      n327 = local read "输入值_2"() -> ()  [unwired: 1 out]
      n328 = local read "输入值_3"() -> ()  [unwired: 1 out]
      n329 = local read "输入值_4"() -> ()  [unwired: 1 out]
      n330 = local read "输入值_5"() -> ()  [unwired: 1 out]
      n331 = local read "输入值_6"() -> ()  [unwired: 1 out]
      n332 = local read "输入值_7"() -> ()  [unwired: 1 out]
      n333 = local read "输入值_8"() -> ()  [unwired: 1 out]
      n334 = local read "输入值_9"() -> ()  [unwired: 1 out]
      n335 = local read "输入值_10"() -> ()  [unwired: 1 out]
      n336 = local read "输入值_11"() -> ()  [unwired: 1 out]
      n337 = local read "输入值_12"() -> ()  [unwired: 1 out]
      n338 = local read "输入值_13"() -> ()  [unwired: 1 out]
      n339 = local read "输入值_14"() -> ()  [unwired: 1 out]
      n340 = local read "输入值_15"() -> ()  [unwired: 1 out]
      n341 = local read "输入值_16"() -> ()  [unwired: 1 out]
      n342 = local read "输入值_17"() -> ()  [unwired: 1 out]
      n343 = local read "输入值_18"() -> ()  [unwired: 1 out]
      n344 = local read "输入值_19"() -> ()  [unwired: 1 out]
      n345 = local read "输入值_20"() -> ()  [unwired: 1 out]
      n346 = local read "输入值_21"() -> ()  [unwired: 1 out]
      n347 = local read "输入值_22"() -> ()  [unwired: 1 out]
      n348 = local read "输入值_23"() -> ()  [unwired: 1 out]
      n349 = local read "输入值_24"() -> ()  [unwired: 1 out]
      n350 = local read "输入值_25"() -> ()  [unwired: 1 out]
      n351 = local read "输入值_26"() -> ()  [unwired: 1 out]
      n352 = local read "输入值_27"() -> ()  [unwired: 1 out]
      n353 = local read "输入值_28"() -> ()  [unwired: 1 out]
      n354 = local read "输入值_29"() -> ()  [unwired: 1 out]
      n355 = local read "输入值_30"() -> ()  [unwired: 1 out]
      n356 = local read "输入值_31"() -> ()  [unwired: 1 out]
      n357 = local read "输入值_32"() -> ()  [unwired: 1 out]
      n358 = local read "输入值_33"() -> ()  [unwired: 1 out]
      n359 = local read "输入值_34"() -> ()  [unwired: 1 out]
      n360 = local read "输入值_35"() -> ()  [unwired: 1 out]
      n361 = local read "输入值_36"() -> ()  [unwired: 1 out]
      n362 = local read "输入值_37"() -> ()  [unwired: 1 out]
      n363 = local read "输入值_38"() -> ()  [unwired: 1 out]
      n364 = local read "输入值_39"() -> ()  [unwired: 1 out]
      n365 = local read "输入值_40"() -> ()  [unwired: 1 out]
      n366 = local read "输入值_41"() -> ()  [unwired: 1 out]
      n367 = local read "输入值_42"() -> ()  [unwired: 1 out]
      n368 = local read "输入值_43"() -> ()  [unwired: 1 out]
      n369 = local read "输入值_44"() -> ()  [unwired: 1 out]
      n370 = local read "输入值_45"() -> ()  [unwired: 1 out]
      n371 = local read "输入值_46"() -> ()  [unwired: 1 out]
      n372 = local read "输入值_47"() -> ()  [unwired: 1 out]
      n373 = local read "输入值_48"() -> ()  [unwired: 1 out]
      n374 = local read "输入值_49"() -> ()  [unwired: 1 out]
      n375 = local read "输入值_50"() -> ()  [unwired: 1 out]
      n376 = local read "输入值_51"() -> ()  [unwired: 1 out]
      n377 = local read "输入值_52"() -> ()  [unwired: 1 out]
      n378 = local read "输入值_53"() -> ()  [unwired: 1 out]
      n379 = local read "输入值_54"() -> ()  [unwired: 1 out]
      n380 = local read "输入值_55"() -> ()  [unwired: 1 out]
      n381 = local read "输入值_56"() -> ()  [unwired: 1 out]
      n382 = local read "输入值_57"() -> ()  [unwired: 1 out]
      n383 = local read "输入值_58"() -> ()  [unwired: 1 out]
      n384 = local read "输入值_59"() -> ()  [unwired: 1 out]
      n385 = local read "输入值_60"() -> ()  [unwired: 1 out]
      n386 = local read "输入值_61"() -> ()  [unwired: 1 out]
      n387 = local read "输入值_62"() -> ()  [unwired: 1 out]
      n388 = local read "输入值_63"() -> ()  [unwired: 1 out]
      n389 = local read "输入值_64"() -> ()  [unwired: 1 out]
      n390 = local read "输入值_65"() -> ()  [unwired: 1 out]
      n391 = local read "输入值_66"() -> ()  [unwired: 1 out]
      n392 = local read "输入值_67"() -> ()  [unwired: 1 out]
      n393 = local read "输入值_68"() -> ()  [unwired: 1 out]
      n394 = local read "输入值_69"() -> ()  [unwired: 1 out]
      n395 = local read "输入值_70"() -> ()  [unwired: 1 out]
      n396 = local read "输入值_71"() -> ()  [unwired: 1 out]
      n397 = local read "输入值_72"() -> ()  [unwired: 1 out]
      n398 = local read "输入值_73"() -> ()  [unwired: 1 out]
      n399 = local read "输入值_74"() -> ()  [unwired: 1 out]
      n400 = local read "输入值_75"() -> ()  [unwired: 1 out]
      n401 = local read "输入值_76"() -> ()  [unwired: 1 out]
      n402 = local read "输入值_77"() -> ()  [unwired: 1 out]
      n403 = local read "输入值_78"() -> ()  [unwired: 1 out]
      n404 = local read "输入值_79"() -> ()  [unwired: 1 out]
      n405 = local read "输入值_80"() -> ()  [unwired: 1 out]
    }
    frame Enabled {
    }
  }
  n406 = Obtain Notifier(name (unnamed)=w5, notification data type=w5) -> (notifier out=w4:refnum<notifier>, error out=w3:errorcluster)  [unwired: 2 in, 1 out]
  n407 = while {
    tunnel: w4 -> [w17]
    tunnel: w3 -> [w16]
    stop <- w18 stop-if-true
    n408 = event shown="[13] \"btn_开始试验\": 值改变" {
      selector: _ -> [_ _ _ _ _ _ _ _ _ _ _ _ _ _ _ _ _ _ _]
      dyn-events: _ -> [_ _ _ _ _ _ _ _ _ _ _ _ _ _ _ _ _ _ _]
      timeout: _ -> [_ _ _ _ _ _ _ _ _ _ _ _ _ _ _ _ _ _ _]
      tunnel: [_ w19 w20 _ _ _ _ _ _ _ _ _ _ _ _ _ _ _ _] -> w18
      tunnel: w17 -> [_ _ _ _ _ _ _ _ _ _ _ _ _ w62 _ _ _ _ _]
      tunnel: w16 -> [_ _ _ _ _ _ _ _ _ _ _ _ _ w61 _ _ _ _ _]
      event Timeout {
        n409 = event-data() -> ()  [unwired: 1 in, 2 out]
      }
      event Panel Close {
        w19 = TRUE ("关闭？")
        n410 = event-data() -> ()  [unwired: 1 in, 3 out]
        n411 = local write "关闭？"(w19) -> ()
      }
      event "btn_关闭": Value Change {
        w20 = TRUE
        n412 = event-data() -> ()  [unwired: 1 in, 5 out]
        n413 = local write "关闭？"(w20) -> ()
      }
      event "btn_全选_1": Value Change {
        n414 = event-data() -> ("NewVal"=w22:bool)  [unwired: 1 in, 4 out]
        n415 = case shown="假" w22 {
          tunnel: [FALSE ("单选_第41路") TRUE ("单选_第41路")] -> w21
          frame False {
          }
          frame True {
          }
        }
        n416 = local write "单选_第1路"(w21) -> ()
        n417 = local write "单选_第2路"(w21) -> ()
        n418 = local write "单选_第3路"(w21) -> ()
        n419 = local write "单选_第4路"(w21) -> ()
        n420 = local write "单选_第5路"(w21) -> ()
        n421 = local write "单选_第6路"(w21) -> ()
        n422 = local write "单选_第7路"(w21) -> ()
        n423 = local write "单选_第8路"(w21) -> ()
        n424 = local write "单选_第9路"(w21) -> ()
        n425 = local write "单选_第10路"(w21) -> ()
        n426 = local write "单选_第11路"(w21) -> ()
        n427 = local write "单选_第12路"(w21) -> ()
        n428 = local write "单选_第13路"(w21) -> ()
        n429 = local write "单选_第14路"(w21) -> ()
        n430 = local write "单选_第15路"(w21) -> ()
        n431 = local write "单选_第16路"(w21) -> ()
      }
      event "btn_全选_2": Value Change {
        n432 = event-data() -> ("NewVal"=w26:bool)  [unwired: 1 in, 4 out]
        n433 = case shown="假" w26 {
          tunnel: [FALSE ("单选_第41路") TRUE ("单选_第41路")] -> w25
          frame False {
          }
          frame True {
          }
        }
        n434 = local write "单选_第17路"(w25) -> ()
        n435 = local write "单选_第18路"(w25) -> ()
        n436 = local write "单选_第19路"(w25) -> ()
        n437 = local write "单选_第20路"(w25) -> ()
        n438 = local write "单选_第21路"(w25) -> ()
        n439 = local write "单选_第22路"(w25) -> ()
        n440 = local write "单选_第23路"(w25) -> ()
        n441 = local write "单选_第24路"(w25) -> ()
        n442 = local write "单选_第25路"(w25) -> ()
        n443 = local write "单选_第26路"(w25) -> ()
        n444 = local write "单选_第27路"(w25) -> ()
        n445 = local write "单选_第28路"(w25) -> ()
        n446 = local write "单选_第29路"(w25) -> ()
        n447 = local write "单选_第30路"(w25) -> ()
        n448 = local write "单选_第31路"(w25) -> ()
        n449 = local write "单选_第32路"(w25) -> ()
      }
      event "btn_全选_3": Value Change {
        n450 = event-data() -> ("NewVal"=w30:bool)  [unwired: 1 in, 4 out]
        n451 = case shown="假" w30 {
          tunnel: [FALSE ("单选_第41路") TRUE ("单选_第41路")] -> w29
          frame False {
          }
          frame True {
          }
        }
        n452 = local write "单选_第33路"(w29) -> ()
        n453 = local write "单选_第34路"(w29) -> ()
        n454 = local write "单选_第35路"(w29) -> ()
        n455 = local write "单选_第36路"(w29) -> ()
        n456 = local write "单选_第37路"(w29) -> ()
        n457 = local write "单选_第38路"(w29) -> ()
        n458 = local write "单选_第39路"(w29) -> ()
        n459 = local write "单选_第40路"(w29) -> ()
        n460 = local write "单选_第41路"(w29) -> ()
        n461 = local write "单选_第42路"(w29) -> ()
        n462 = local write "单选_第43路"(w29) -> ()
        n463 = local write "单选_第44路"(w29) -> ()
        n464 = local write "单选_第45路"(w29) -> ()
        n465 = local write "单选_第46路"(w29) -> ()
        n466 = local write "单选_第47路"(w29) -> ()
        n467 = local write "单选_第48路"(w29) -> ()
      }
      event "btn_全选_4": Value Change {
        n468 = event-data() -> ("NewVal"=w34:bool)  [unwired: 1 in, 4 out]
        n469 = case shown="假" w34 {
          tunnel: [FALSE ("单选_第41路") TRUE ("单选_第41路")] -> w33
          frame False {
          }
          frame True {
          }
        }
        n470 = local write "单选_第49路"(w33) -> ()
        n471 = local write "单选_第50路"(w33) -> ()
        n472 = local write "单选_第51路"(w33) -> ()
        n473 = local write "单选_第52路"(w33) -> ()
        n474 = local write "单选_第53路"(w33) -> ()
        n475 = local write "单选_第54路"(w33) -> ()
        n476 = local write "单选_第55路"(w33) -> ()
        n477 = local write "单选_第56路"(w33) -> ()
        n478 = local write "单选_第57路"(w33) -> ()
        n479 = local write "单选_第58路"(w33) -> ()
        n480 = local write "单选_第59路"(w33) -> ()
        n481 = local write "单选_第60路"(w33) -> ()
        n482 = local write "单选_第61路"(w33) -> ()
        n483 = local write "单选_第62路"(w33) -> ()
        n484 = local write "单选_第63路"(w33) -> ()
        n485 = local write "单选_第64路"(w33) -> ()
      }
      event "btn_全选_5": Value Change {
        n486 = event-data() -> ("NewVal"=w38:bool)  [unwired: 1 in, 4 out]
        n487 = case shown="假" w38 {
          tunnel: [FALSE ("单选_第41路") TRUE ("单选_第41路")] -> w37
          frame False {
          }
          frame True {
          }
        }
        n488 = local write "单选_第71路"(w37) -> ()
        n489 = local write "单选_第79路"(w37) -> ()
        n490 = local write "单选_第65路"(w37) -> ()
        n491 = local write "单选_第66路"(w37) -> ()
        n492 = local write "单选_第67路"(w37) -> ()
        n493 = local write "单选_第68路"(w37) -> ()
        n494 = local write "单选_第69路"(w37) -> ()
        n495 = local write "单选_第70路"(w37) -> ()
        n496 = local write "单选_第72路"(w37) -> ()
        n497 = local write "单选_第73路"(w37) -> ()
        n498 = local write "单选_第74路"(w37) -> ()
        n499 = local write "单选_第75路"(w37) -> ()
        n500 = local write "单选_第76路"(w37) -> ()
        n501 = local write "单选_第77路"(w37) -> ()
        n502 = local write "单选_第78路"(w37) -> ()
        n503 = local write "单选_第80路"(w37) -> ()
      }
      event "btn_置1_1": Value Change {
        n504 = event-data() -> ("NewVal"=w42:bool)  [unwired: 1 in, 4 out]
        n505 = case shown="假" w42 {
          tunnel: [enum16{"0", "1"}."0" ("输入值_41") enum16{"0", "1"}."1" ("输入值_41")] -> w41
          frame False {
          }
          frame True {
          }
        }
        n506 = local write "输入值_1"(w41) -> ()
        n507 = local write "输入值_2"(w41) -> ()
        n508 = local write "输入值_3"(w41) -> ()
        n509 = local write "输入值_4"(w41) -> ()
        n510 = local write "输入值_5"(w41) -> ()
        n511 = local write "输入值_6"(w41) -> ()
        n512 = local write "输入值_7"(w41) -> ()
        n513 = local write "输入值_8"(w41) -> ()
        n514 = local write "输入值_9"(w41) -> ()
        n515 = local write "输入值_10"(w41) -> ()
        n516 = local write "输入值_11"(w41) -> ()
        n517 = local write "输入值_12"(w41) -> ()
        n518 = local write "输入值_13"(w41) -> ()
        n519 = local write "输入值_14"(w41) -> ()
        n520 = local write "输入值_15"(w41) -> ()
        n521 = local write "输入值_16"(w41) -> ()
      }
      event "btn_置1_2": Value Change {
        n522 = event-data() -> ("NewVal"=w46:bool)  [unwired: 1 in, 4 out]
        n523 = case shown="假" w46 {
          tunnel: [enum16{"0", "1"}."0" ("输入值_41") enum16{"0", "1"}."1" ("输入值_41")] -> w45
          frame False {
          }
          frame True {
          }
        }
        n524 = local write "输入值_17"(w45) -> ()
        n525 = local write "输入值_18"(w45) -> ()
        n526 = local write "输入值_19"(w45) -> ()
        n527 = local write "输入值_20"(w45) -> ()
        n528 = local write "输入值_21"(w45) -> ()
        n529 = local write "输入值_22"(w45) -> ()
        n530 = local write "输入值_23"(w45) -> ()
        n531 = local write "输入值_24"(w45) -> ()
        n532 = local write "输入值_25"(w45) -> ()
        n533 = local write "输入值_26"(w45) -> ()
        n534 = local write "输入值_27"(w45) -> ()
        n535 = local write "输入值_28"(w45) -> ()
        n536 = local write "输入值_29"(w45) -> ()
        n537 = local write "输入值_30"(w45) -> ()
        n538 = local write "输入值_31"(w45) -> ()
        n539 = local write "输入值_32"(w45) -> ()
      }
      event "btn_置1_3": Value Change {
        n540 = event-data() -> ("NewVal"=w50:bool)  [unwired: 1 in, 4 out]
        n541 = case shown="假" w50 {
          tunnel: [enum16{"0", "1"}."0" ("输入值_41") enum16{"0", "1"}."1" ("输入值_41")] -> w49
          frame False {
          }
          frame True {
          }
        }
        n542 = local write "输入值_33"(w49) -> ()
        n543 = local write "输入值_34"(w49) -> ()
        n544 = local write "输入值_35"(w49) -> ()
        n545 = local write "输入值_36"(w49) -> ()
        n546 = local write "输入值_37"(w49) -> ()
        n547 = local write "输入值_38"(w49) -> ()
        n548 = local write "输入值_39"(w49) -> ()
        n549 = local write "输入值_40"(w49) -> ()
        n550 = local write "输入值_41"(w49) -> ()
        n551 = local write "输入值_42"(w49) -> ()
        n552 = local write "输入值_43"(w49) -> ()
        n553 = local write "输入值_44"(w49) -> ()
        n554 = local write "输入值_45"(w49) -> ()
        n555 = local write "输入值_46"(w49) -> ()
        n556 = local write "输入值_47"(w49) -> ()
        n557 = local write "输入值_48"(w49) -> ()
      }
      event "btn_置1_4": Value Change {
        n558 = event-data() -> ("NewVal"=w54:bool)  [unwired: 1 in, 4 out]
        n559 = case shown="假" w54 {
          tunnel: [enum16{"0", "1"}."0" ("输入值_41") enum16{"0", "1"}."1" ("输入值_41")] -> w53
          frame False {
          }
          frame True {
          }
        }
        n560 = local write "输入值_49"(w53) -> ()
        n561 = local write "输入值_50"(w53) -> ()
        n562 = local write "输入值_51"(w53) -> ()
        n563 = local write "输入值_52"(w53) -> ()
        n564 = local write "输入值_53"(w53) -> ()
        n565 = local write "输入值_54"(w53) -> ()
        n566 = local write "输入值_55"(w53) -> ()
        n567 = local write "输入值_56"(w53) -> ()
        n568 = local write "输入值_57"(w53) -> ()
        n569 = local write "输入值_58"(w53) -> ()
        n570 = local write "输入值_59"(w53) -> ()
        n571 = local write "输入值_60"(w53) -> ()
        n572 = local write "输入值_61"(w53) -> ()
        n573 = local write "输入值_62"(w53) -> ()
        n574 = local write "输入值_63"(w53) -> ()
        n575 = local write "输入值_64"(w53) -> ()
      }
      event "btn_置1_5": Value Change {
        n576 = event-data() -> ("NewVal"=w58:bool)  [unwired: 1 in, 4 out]
        n577 = case shown="假" w58 {
          tunnel: [enum16{"0", "1"}."0" ("输入值_41") enum16{"0", "1"}."1" ("输入值_41")] -> w57
          frame False {
          }
          frame True {
          }
        }
        n578 = local write "输入值_65"(w57) -> ()
        n579 = local write "输入值_66"(w57) -> ()
        n580 = local write "输入值_67"(w57) -> ()
        n581 = local write "输入值_68"(w57) -> ()
        n582 = local write "输入值_69"(w57) -> ()
        n583 = local write "输入值_70"(w57) -> ()
        n584 = local write "输入值_71"(w57) -> ()
        n585 = local write "输入值_72"(w57) -> ()
        n586 = local write "输入值_73"(w57) -> ()
        n587 = local write "输入值_74"(w57) -> ()
        n588 = local write "输入值_75"(w57) -> ()
        n589 = local write "输入值_76"(w57) -> ()
        n590 = local write "输入值_77"(w57) -> ()
        n591 = local write "输入值_78"(w57) -> ()
        n592 = local write "输入值_79"(w57) -> ()
        n593 = local write "输入值_80"(w57) -> ()
      }
      event "btn_开始试验": Value Change {
        n594 = event-data() -> ()  [unwired: 1 in, 5 out]
        n595 = stacked-sequence {
          tunnel: w62 -> [_ _ _ w299]
          tunnel: w61 -> [_ _ _ w298]
          frame #0 {
            w67 = 0 ("同步_A2")
            n596 = stacked-sequence {
              tunnel: [w91 _ _ _ _] -> w87
              tunnel: [w90 _ _ _ _] -> w72
              tunnel: [_ w125 _ _ _] -> w85
              tunnel: [_ w124 _ _ _] -> w71
              tunnel: [_ _ w159 _ _] -> w83
              tunnel: [_ _ w158 _ _] -> w70
              tunnel: [_ _ _ w193 _] -> w81
              tunnel: [_ _ _ w192 _] -> w69
              tunnel: [_ _ _ _ w227] -> w63
              tunnel: [_ _ _ _ w226] -> w65
              frame #0 {
                n597 = local read "单选_第1路"() -> (w108:bool)
                n598 = local read "单选_第2路"() -> (w109:bool)
                n599 = local read "单选_第3路"() -> (w110:bool)
                n600 = local read "单选_第4路"() -> (w111:bool)
                n601 = local read "单选_第5路"() -> (w112:bool)
                n602 = local read "单选_第6路"() -> (w113:bool)
                n603 = local read "单选_第7路"() -> (w114:bool)
                n604 = local read "单选_第8路"() -> (w115:bool)
                n605 = local read "单选_第9路"() -> (w116:bool)
                n606 = local read "单选_第10路"() -> (w117:bool)
                n607 = local read "单选_第11路"() -> (w118:bool)
                n608 = local read "单选_第12路"() -> (w119:bool)
                n609 = local read "单选_第13路"() -> (w120:bool)
                n610 = local read "单选_第14路"() -> (w121:bool)
                n611 = local read "单选_第15路"() -> (w122:bool)
                n612 = local read "单选_第16路"() -> (w123:bool)
                n613 = local read "输入值_1"() -> (w92:enum16{"0", "1"})
                n614 = local read "输入值_2"() -> (w93:enum16{"0", "1"})
                n615 = local read "输入值_3"() -> (w94:enum16{"0", "1"})
                n616 = local read "输入值_4"() -> (w95:enum16{"0", "1"})
                n617 = local read "输入值_5"() -> (w96:enum16{"0", "1"})
                n618 = local read "输入值_6"() -> (w97:enum16{"0", "1"})
                n619 = local read "输入值_7"() -> (w98:enum16{"0", "1"})
                n620 = local read "输入值_8"() -> (w99:enum16{"0", "1"})
                n621 = local read "输入值_9"() -> (w100:enum16{"0", "1"})
                n622 = local read "输入值_10"() -> (w101:enum16{"0", "1"})
                n623 = local read "输入值_11"() -> (w102:enum16{"0", "1"})
                n624 = local read "输入值_12"() -> (w103:enum16{"0", "1"})
                n625 = local read "输入值_13"() -> (w104:enum16{"0", "1"})
                n626 = local read "输入值_14"() -> (w105:enum16{"0", "1"})
                n627 = local read "输入值_15"() -> (w106:enum16{"0", "1"})
                n628 = local read "输入值_16"() -> (w107:enum16{"0", "1"})
                n629 = Build Array(w108, w109, w110, w111, w112, w113, w114, w115, w116, w117, w118, w119, w120, w121, w122, w123) -> (w91:bool[])
                n630 = Build Array(w92, w93, w94, w95, w96, w97, w98, w99, w100, w101, w102, w103, w104, w105, w106, w107) -> (w90:enum16{"0", "1"}[])
              }
              frame #1 {
                n631 = local read "单选_第17路"() -> (w142:bool)
                n632 = local read "单选_第18路"() -> (w143:bool)
                n633 = local read "单选_第19路"() -> (w144:bool)
                n634 = local read "单选_第20路"() -> (w145:bool)
                n635 = local read "单选_第21路"() -> (w146:bool)
                n636 = local read "单选_第22路"() -> (w147:bool)
                n637 = local read "单选_第23路"() -> (w148:bool)
                n638 = local read "单选_第24路"() -> (w149:bool)
                n639 = local read "单选_第25路"() -> (w150:bool)
                n640 = local read "单选_第26路"() -> (w151:bool)
                n641 = local read "单选_第27路"() -> (w152:bool)
                n642 = local read "单选_第28路"() -> (w153:bool)
                n643 = local read "单选_第29路"() -> (w154:bool)
                n644 = local read "单选_第30路"() -> (w155:bool)
                n645 = local read "单选_第31路"() -> (w156:bool)
                n646 = local read "单选_第32路"() -> (w157:bool)
                n647 = local read "输入值_17"() -> (w126:enum16{"0", "1"})
                n648 = local read "输入值_18"() -> (w127:enum16{"0", "1"})
                n649 = local read "输入值_19"() -> (w128:enum16{"0", "1"})
                n650 = local read "输入值_20"() -> (w129:enum16{"0", "1"})
                n651 = local read "输入值_21"() -> (w130:enum16{"0", "1"})
                n652 = local read "输入值_22"() -> (w131:enum16{"0", "1"})
                n653 = local read "输入值_23"() -> (w132:enum16{"0", "1"})
                n654 = local read "输入值_24"() -> (w133:enum16{"0", "1"})
                n655 = local read "输入值_25"() -> (w134:enum16{"0", "1"})
                n656 = local read "输入值_26"() -> (w135:enum16{"0", "1"})
                n657 = local read "输入值_27"() -> (w136:enum16{"0", "1"})
                n658 = local read "输入值_28"() -> (w137:enum16{"0", "1"})
                n659 = local read "输入值_29"() -> (w138:enum16{"0", "1"})
                n660 = local read "输入值_30"() -> (w139:enum16{"0", "1"})
                n661 = local read "输入值_31"() -> (w140:enum16{"0", "1"})
                n662 = local read "输入值_32"() -> (w141:enum16{"0", "1"})
                n663 = Build Array(w142, w143, w144, w145, w146, w147, w148, w149, w150, w151, w152, w153, w154, w155, w156, w157) -> (w125:bool[])
                n664 = Build Array(w126, w127, w128, w129, w130, w131, w132, w133, w134, w135, w136, w137, w138, w139, w140, w141) -> (w124:enum16{"0", "1"}[])
              }
              frame #2 {
                n665 = local read "单选_第33路"() -> (w176:bool)
                n666 = local read "单选_第34路"() -> (w177:bool)
                n667 = local read "单选_第35路"() -> (w178:bool)
                n668 = local read "单选_第36路"() -> (w179:bool)
                n669 = local read "单选_第37路"() -> (w180:bool)
                n670 = local read "单选_第38路"() -> (w181:bool)
                n671 = local read "单选_第39路"() -> (w182:bool)
                n672 = local read "单选_第40路"() -> (w183:bool)
                n673 = local read "单选_第41路"() -> (w184:bool)
                n674 = local read "单选_第42路"() -> (w185:bool)
                n675 = local read "单选_第43路"() -> (w186:bool)
                n676 = local read "单选_第44路"() -> (w187:bool)
                n677 = local read "单选_第45路"() -> (w188:bool)
                n678 = local read "单选_第46路"() -> (w189:bool)
                n679 = local read "单选_第47路"() -> (w190:bool)
                n680 = local read "单选_第48路"() -> (w191:bool)
                n681 = local read "输入值_33"() -> (w160:enum16{"0", "1"})
                n682 = local read "输入值_34"() -> (w161:enum16{"0", "1"})
                n683 = local read "输入值_35"() -> (w162:enum16{"0", "1"})
                n684 = local read "输入值_36"() -> (w163:enum16{"0", "1"})
                n685 = local read "输入值_37"() -> (w164:enum16{"0", "1"})
                n686 = local read "输入值_38"() -> (w165:enum16{"0", "1"})
                n687 = local read "输入值_39"() -> (w166:enum16{"0", "1"})
                n688 = local read "输入值_40"() -> (w167:enum16{"0", "1"})
                n689 = local read "输入值_41"() -> (w168:enum16{"0", "1"})
                n690 = local read "输入值_42"() -> (w169:enum16{"0", "1"})
                n691 = local read "输入值_43"() -> (w170:enum16{"0", "1"})
                n692 = local read "输入值_44"() -> (w171:enum16{"0", "1"})
                n693 = local read "输入值_45"() -> (w172:enum16{"0", "1"})
                n694 = local read "输入值_46"() -> (w173:enum16{"0", "1"})
                n695 = local read "输入值_47"() -> (w174:enum16{"0", "1"})
                n696 = local read "输入值_48"() -> (w175:enum16{"0", "1"})
                n697 = Build Array(w160, w161, w162, w163, w164, w165, w166, w167, w168, w169, w170, w171, w172, w173, w174, w175) -> (w158:enum16{"0", "1"}[])
                n698 = Build Array(w176, w177, w178, w179, w180, w181, w182, w183, w184, w185, w186, w187, w188, w189, w190, w191) -> (w159:bool[])
              }
              frame #3 {
                n699 = local read "单选_第49路"() -> (w210:bool)
                n700 = local read "单选_第50路"() -> (w211:bool)
                n701 = local read "单选_第51路"() -> (w212:bool)
                n702 = local read "单选_第52路"() -> (w213:bool)
                n703 = local read "单选_第53路"() -> (w214:bool)
                n704 = local read "单选_第54路"() -> (w215:bool)
                n705 = local read "单选_第55路"() -> (w216:bool)
                n706 = local read "单选_第56路"() -> (w217:bool)
                n707 = local read "单选_第57路"() -> (w218:bool)
                n708 = local read "单选_第58路"() -> (w219:bool)
                n709 = local read "单选_第59路"() -> (w220:bool)
                n710 = local read "单选_第60路"() -> (w221:bool)
                n711 = local read "单选_第61路"() -> (w222:bool)
                n712 = local read "单选_第62路"() -> (w223:bool)
                n713 = local read "单选_第63路"() -> (w224:bool)
                n714 = local read "单选_第64路"() -> (w225:bool)
                n715 = local read "输入值_49"() -> (w194:enum16{"0", "1"})
                n716 = local read "输入值_50"() -> (w195:enum16{"0", "1"})
                n717 = local read "输入值_51"() -> (w196:enum16{"0", "1"})
                n718 = local read "输入值_52"() -> (w197:enum16{"0", "1"})
                n719 = local read "输入值_53"() -> (w198:enum16{"0", "1"})
                n720 = local read "输入值_54"() -> (w199:enum16{"0", "1"})
                n721 = local read "输入值_55"() -> (w200:enum16{"0", "1"})
                n722 = local read "输入值_56"() -> (w201:enum16{"0", "1"})
                n723 = local read "输入值_57"() -> (w202:enum16{"0", "1"})
                n724 = local read "输入值_58"() -> (w203:enum16{"0", "1"})
                n725 = local read "输入值_59"() -> (w204:enum16{"0", "1"})
                n726 = local read "输入值_60"() -> (w205:enum16{"0", "1"})
                n727 = local read "输入值_61"() -> (w206:enum16{"0", "1"})
                n728 = local read "输入值_62"() -> (w207:enum16{"0", "1"})
                n729 = local read "输入值_63"() -> (w208:enum16{"0", "1"})
                n730 = local read "输入值_64"() -> (w209:enum16{"0", "1"})
                n731 = Build Array(w210, w211, w212, w213, w214, w215, w216, w217, w218, w219, w220, w221, w222, w223, w224, w225) -> (w193:bool[])
                n732 = Build Array(w194, w195, w196, w197, w198, w199, w200, w201, w202, w203, w204, w205, w206, w207, w208, w209) -> (w192:enum16{"0", "1"}[])
              }
              frame #4 {
                n733 = local read "单选_第71路"() -> (w250:bool)
                n734 = local read "单选_第79路"() -> (w258:bool)
                n735 = local read "单选_第65路"() -> (w244:bool)
                n736 = local read "单选_第66路"() -> (w245:bool)
                n737 = local read "单选_第67路"() -> (w246:bool)
                n738 = local read "单选_第68路"() -> (w247:bool)
                n739 = local read "单选_第69路"() -> (w248:bool)
                n740 = local read "单选_第70路"() -> (w249:bool)
                n741 = local read "单选_第72路"() -> (w251:bool)
                n742 = local read "单选_第73路"() -> (w252:bool)
                n743 = local read "单选_第74路"() -> (w253:bool)
                n744 = local read "单选_第75路"() -> (w254:bool)
                n745 = local read "单选_第76路"() -> (w255:bool)
                n746 = local read "单选_第77路"() -> (w256:bool)
                n747 = local read "单选_第78路"() -> (w257:bool)
                n748 = local read "单选_第80路"() -> (w259:bool)
                n749 = local read "输入值_65"() -> (w228:enum16{"0", "1"})
                n750 = local read "输入值_66"() -> (w229:enum16{"0", "1"})
                n751 = local read "输入值_67"() -> (w230:enum16{"0", "1"})
                n752 = local read "输入值_68"() -> (w231:enum16{"0", "1"})
                n753 = local read "输入值_69"() -> (w232:enum16{"0", "1"})
                n754 = local read "输入值_70"() -> (w233:enum16{"0", "1"})
                n755 = local read "输入值_71"() -> (w234:enum16{"0", "1"})
                n756 = local read "输入值_72"() -> (w235:enum16{"0", "1"})
                n757 = local read "输入值_73"() -> (w236:enum16{"0", "1"})
                n758 = local read "输入值_74"() -> (w237:enum16{"0", "1"})
                n759 = local read "输入值_75"() -> (w238:enum16{"0", "1"})
                n760 = local read "输入值_76"() -> (w239:enum16{"0", "1"})
                n761 = local read "输入值_77"() -> (w240:enum16{"0", "1"})
                n762 = local read "输入值_78"() -> (w241:enum16{"0", "1"})
                n763 = local read "输入值_79"() -> (w242:enum16{"0", "1"})
                n764 = local read "输入值_80"() -> (w243:enum16{"0", "1"})
                n765 = Build Array(w228, w229, w230, w231, w232, w233, w234, w235, w236, w237, w238, w239, w240, w241, w242, w243) -> (w226:enum16{"0", "1"}[])
                n766 = Build Array(w244, w245, w246, w247, w248, w249, w250, w251, w252, w253, w254, w255, w256, w257, w258, w259) -> (w227:bool[])
              }
            }
            n767 = local read "数组_选择?"() -> (w89:bool[][])
            n768 = local read "数组_输入值"() -> (w73:enum16{"0", "1"}[][])
            n769 = Replace Array Subset(array=w89, new element #1=w87, index (row) #1=0 ("索引 (行)"), new element #2=w85, index (row) #2=1 ("索引 (行)"), new element #3=w83, index (row) #3=2 ("索引 (行)"), new element #4=w81, index (row) #4=3 ("索引 (行)"), new element #5=w63, index (row) #5=4 ("索引 (行)"), new element #6=w63, index (row) #6=5 ("索引 (行)")) -> (w79:bool[][])  [unwired: 6 in]
            n770 = Replace Array Subset(array=w73, new element #1=w72, index (row) #1=0 ("索引 (行)"), new element #2=w71, index (row) #2=1 ("索引 (行)"), new element #3=w70, index (row) #3=2 ("索引 (行)"), new element #4=w69, index (row) #4=3 ("索引 (行)"), new element #5=w65, index (row) #5=4 ("索引 (行)"), new element #6=w65, index (row) #6=5 ("索引 (行)")) -> (w68:enum16{"0", "1"}[][])  [unwired: 6 in]
            n771 = local write "数组_选择?"(w79) -> ()
            n772 = local write "数组_输入值"(w68) -> ()
            n773 = local write "同步_A2"(w67) -> ()
            n774 = local write "同步_A1"(w67) -> ()
          }
          frame #1 {
            w264 = cluster{u32, u32}[] [{9868950, 9868950}]
            n775 = property on="light_1" class="Bool (严格)"("Colors [4]"=w264) -> ()  [unwired: 2 in, 2 out]
            n776 = property on="light_2" class="Bool (严格)"("Colors [4]"=w264) -> ()  [unwired: 2 in, 2 out]
            n777 = property on="light_3" class="Bool (严格)"("Colors [4]"=w264) -> ()  [unwired: 2 in, 2 out]
            n778 = property on="light_4" class="Bool (严格)"("Colors [4]"=w264) -> ()  [unwired: 2 in, 2 out]
            n779 = property on="light_5" class="Bool (严格)"("Colors [4]"=w264) -> ()  [unwired: 2 in, 2 out]
            n780 = property on="light_6" class="Bool (严格)"("Colors [4]"=w264) -> ()  [unwired: 2 in, 2 out]
            n781 = property on="light_7" class="Bool (严格)"("Colors [4]"=w264) -> ()  [unwired: 2 in, 2 out]
            n782 = property on="light_8" class="Bool (严格)"("Colors [4]"=w264) -> ()  [unwired: 2 in, 2 out]
            n783 = property on="light_9" class="Bool (严格)"("Colors [4]"=w264) -> ()  [unwired: 2 in, 2 out]
            n784 = property on="light_10" class="Bool (严格)"("Colors [4]"=w264) -> ()  [unwired: 2 in, 2 out]
            n785 = property on="light_11" class="Bool (严格)"("Colors [4]"=w264) -> ()  [unwired: 2 in, 2 out]
            n786 = property on="light_12" class="Bool (严格)"("Colors [4]"=w264) -> ()  [unwired: 2 in, 2 out]
            n787 = property on="light_13" class="Bool (严格)"("Colors [4]"=w264) -> ()  [unwired: 2 in, 2 out]
            n788 = property on="light_14" class="Bool (严格)"("Colors [4]"=w264) -> ()  [unwired: 2 in, 2 out]
            n789 = property on="light_15" class="Bool (严格)"("Colors [4]"=w264) -> ()  [unwired: 2 in, 2 out]
            n790 = property on="light_16" class="Bool (严格)"("Colors [4]"=w264) -> ()  [unwired: 2 in, 2 out]
            n791 = property on="light_17" class="Bool (严格)"("Colors [4]"=w264) -> ()  [unwired: 2 in, 2 out]
            n792 = property on="light_18" class="Bool (严格)"("Colors [4]"=w264) -> ()  [unwired: 2 in, 2 out]
            n793 = property on="light_19" class="Bool (严格)"("Colors [4]"=w264) -> ()  [unwired: 2 in, 2 out]
            n794 = property on="light_20" class="Bool (严格)"("Colors [4]"=w264) -> ()  [unwired: 2 in, 2 out]
            n795 = property on="light_21" class="Bool (严格)"("Colors [4]"=w264) -> ()  [unwired: 2 in, 2 out]
            n796 = property on="light_22" class="Bool (严格)"("Colors [4]"=w264) -> ()  [unwired: 2 in, 2 out]
            n797 = property on="light_23" class="Bool (严格)"("Colors [4]"=w264) -> ()  [unwired: 2 in, 2 out]
            n798 = property on="light_24" class="Bool (严格)"("Colors [4]"=w264) -> ()  [unwired: 2 in, 2 out]
            n799 = property on="light_25" class="Bool (严格)"("Colors [4]"=w264) -> ()  [unwired: 2 in, 2 out]
            n800 = property on="light_26" class="Bool (严格)"("Colors [4]"=w264) -> ()  [unwired: 2 in, 2 out]
            n801 = property on="light_27" class="Bool (严格)"("Colors [4]"=w264) -> ()  [unwired: 2 in, 2 out]
            n802 = property on="light_28" class="Bool (严格)"("Colors [4]"=w264) -> ()  [unwired: 2 in, 2 out]
            n803 = property on="light_29" class="Bool (严格)"("Colors [4]"=w264) -> ()  [unwired: 2 in, 2 out]
            n804 = property on="light_30" class="Bool (严格)"("Colors [4]"=w264) -> ()  [unwired: 2 in, 2 out]
            n805 = property on="light_31" class="Bool (严格)"("Colors [4]"=w264) -> ()  [unwired: 2 in, 2 out]
            n806 = property on="light_32" class="Bool (严格)"("Colors [4]"=w264) -> ()  [unwired: 2 in, 2 out]
            n807 = property on="light_33" class="Bool (严格)"("Colors [4]"=w264) -> ()  [unwired: 2 in, 2 out]
            n808 = property on="light_34" class="Bool (严格)"("Colors [4]"=w264) -> ()  [unwired: 2 in, 2 out]
            n809 = property on="light_35" class="Bool (严格)"("Colors [4]"=w264) -> ()  [unwired: 2 in, 2 out]
            n810 = property on="light_36" class="Bool (严格)"("Colors [4]"=w264) -> ()  [unwired: 2 in, 2 out]
            n811 = property on="light_37" class="Bool (严格)"("Colors [4]"=w264) -> ()  [unwired: 2 in, 2 out]
            n812 = property on="light_38" class="Bool (严格)"("Colors [4]"=w264) -> ()  [unwired: 2 in, 2 out]
            n813 = property on="light_39" class="Bool (严格)"("Colors [4]"=w264) -> ()  [unwired: 2 in, 2 out]
            n814 = property on="light_40" class="Bool (严格)"("Colors [4]"=w264) -> ()  [unwired: 2 in, 2 out]
            n815 = property on="light_41" class="Bool (严格)"("Colors [4]"=w264) -> ()  [unwired: 2 in, 2 out]
            n816 = property on="light_42" class="Bool (严格)"("Colors [4]"=w264) -> ()  [unwired: 2 in, 2 out]
            n817 = property on="light_43" class="Bool (严格)"("Colors [4]"=w264) -> ()  [unwired: 2 in, 2 out]
            n818 = property on="light_44" class="Bool (严格)"("Colors [4]"=w264) -> ()  [unwired: 2 in, 2 out]
            n819 = property on="light_45" class="Bool (严格)"("Colors [4]"=w264) -> ()  [unwired: 2 in, 2 out]
            n820 = property on="light_46" class="Bool (严格)"("Colors [4]"=w264) -> ()  [unwired: 2 in, 2 out]
            n821 = property on="light_47" class="Bool (严格)"("Colors [4]"=w264) -> ()  [unwired: 2 in, 2 out]
            n822 = property on="light_48" class="Bool (严格)"("Colors [4]"=w264) -> ()  [unwired: 2 in, 2 out]
            n823 = property on="light_49" class="Bool (严格)"("Colors [4]"=w264) -> ()  [unwired: 2 in, 2 out]
            n824 = property on="light_50" class="Bool (严格)"("Colors [4]"=w264) -> ()  [unwired: 2 in, 2 out]
            n825 = property on="light_51" class="Bool (严格)"("Colors [4]"=w264) -> ()  [unwired: 2 in, 2 out]
            n826 = property on="light_52" class="Bool (严格)"("Colors [4]"=w264) -> ()  [unwired: 2 in, 2 out]
            n827 = property on="light_53" class="Bool (严格)"("Colors [4]"=w264) -> ()  [unwired: 2 in, 2 out]
            n828 = property on="light_54" class="Bool (严格)"("Colors [4]"=w264) -> ()  [unwired: 2 in, 2 out]
            n829 = property on="light_55" class="Bool (严格)"("Colors [4]"=w264) -> ()  [unwired: 2 in, 2 out]
            n830 = property on="light_56" class="Bool (严格)"("Colors [4]"=w264) -> ()  [unwired: 2 in, 2 out]
            n831 = property on="light_57" class="Bool (严格)"("Colors [4]"=w264) -> ()  [unwired: 2 in, 2 out]
            n832 = property on="light_58" class="Bool (严格)"("Colors [4]"=w264) -> ()  [unwired: 2 in, 2 out]
            n833 = property on="light_59" class="Bool (严格)"("Colors [4]"=w264) -> ()  [unwired: 2 in, 2 out]
            n834 = property on="light_60" class="Bool (严格)"("Colors [4]"=w264) -> ()  [unwired: 2 in, 2 out]
            n835 = property on="light_61" class="Bool (严格)"("Colors [4]"=w264) -> ()  [unwired: 2 in, 2 out]
            n836 = property on="light_62" class="Bool (严格)"("Colors [4]"=w264) -> ()  [unwired: 2 in, 2 out]
            n837 = property on="light_63" class="Bool (严格)"("Colors [4]"=w264) -> ()  [unwired: 2 in, 2 out]
            n838 = property on="light_64" class="Bool (严格)"("Colors [4]"=w264) -> ()  [unwired: 2 in, 2 out]
            n839 = property on="light_65" class="Bool (严格)"("Colors [4]"=w264) -> ()  [unwired: 2 in, 2 out]
            n840 = property on="light_66" class="Bool (严格)"("Colors [4]"=w264) -> ()  [unwired: 2 in, 2 out]
            n841 = property on="light_67" class="Bool (严格)"("Colors [4]"=w264) -> ()  [unwired: 2 in, 2 out]
            n842 = property on="light_68" class="Bool (严格)"("Colors [4]"=w264) -> ()  [unwired: 2 in, 2 out]
            n843 = property on="light_69" class="Bool (严格)"("Colors [4]"=w264) -> ()  [unwired: 2 in, 2 out]
            n844 = property on="light_70" class="Bool (严格)"("Colors [4]"=w264) -> ()  [unwired: 2 in, 2 out]
            n845 = property on="light_71" class="Bool (严格)"("Colors [4]"=w264) -> ()  [unwired: 2 in, 2 out]
            n846 = property on="light_72" class="Bool (严格)"("Colors [4]"=w264) -> ()  [unwired: 2 in, 2 out]
            n847 = property on="light_73" class="Bool (严格)"("Colors [4]"=w264) -> ()  [unwired: 2 in, 2 out]
            n848 = property on="light_74" class="Bool (严格)"("Colors [4]"=w264) -> ()  [unwired: 2 in, 2 out]
            n849 = property on="light_75" class="Bool (严格)"("Colors [4]"=w264) -> ()  [unwired: 2 in, 2 out]
            n850 = property on="light_76" class="Bool (严格)"("Colors [4]"=w264) -> ()  [unwired: 2 in, 2 out]
            n851 = property on="light_77" class="Bool (严格)"("Colors [4]"=w264) -> ()  [unwired: 2 in, 2 out]
            n852 = property on="light_78" class="Bool (严格)"("Colors [4]"=w264) -> ()  [unwired: 2 in, 2 out]
            n853 = property on="light_79" class="Bool (严格)"("Colors [4]"=w264) -> ()  [unwired: 2 in, 2 out]
            n854 = property on="light_80" class="Bool (严格)"("Colors [4]"=w264) -> ()  [unwired: 2 in, 2 out]
            n855 = Initialize Array("", 16 ("维数大小"), 4 ("维数大小")) -> (w263:string[][])
            n856 = local write "D_IN_1"(w263) -> ()
            n857 = local write "D_IN_2"(w263) -> ()
            n858 = local write "D_IN_3"(w263) -> ()
            n859 = local write "D_IN_4"(w263) -> ()
            n860 = local write "D_IN_5"(w263) -> ()
          }
          frame #2 {
            n861 = local read "保持输入"() -> (w265:bool)
            n862 = case shown="假" w265 {
              frame False {
                n863 = property on="保持输入" class="Bool (严格)"("DisabledEnum"=T1."Disabled and Grayed Out" ("禁用")) -> ()  [unwired: 2 in, 2 out]
              }
              frame True {
                n864 = local read "数组_选择?"() -> (w267:bool[][])
                n865 = for {
                  tunnel: w267 -> [w271] mode=indexing
                  i -> [w269]
                  stop <- w268 stop-if-true
                  n866 = Or Array Elements(Boolean array=w271) -> (logical OR=w270:bool)
                  n867 = case shown="真" w270 {
                    tunnel: w269 -> [_ w273]
                    tunnel: [FALSE w276] -> w268
                    frame False {
                    }
                    frame True {
                      n868 = local write "同步_A1"(w273) -> ()
                      n869 = Increment(x=w273) -> (x+1=w278:i32)
                      n870 = Format Into String(format string="保持第%d组数据输入" ("格式字符串"), w278) -> (resulting string=w279:string)  [unwired: 2 in, 1 out]
                      n871 = call "显示对话框信息2"("Message"=w279) -> ("是"=w274:bool)  [unwired: 9 in, 1 out]
                      n872 = case shown="真" w274 {
                        tunnel: [FALSE w284] -> w276
                        tunnel: [T1."Enabled" ("禁用") w283] -> w275
                        tunnel: w273 -> [_ w282]
                        frame False {
                        }
                        frame True {
                          n873 = stacked-sequence {
                            tunnel: [_ TRUE] -> w284
                            tunnel: [_ T1."Disabled and Grayed Out" ("禁用")] -> w283
                            tunnel: w282 -> [w285 _]
                            frame #0 {
                              n874 = for {
                                N: 5 -> [_]
                                tunnel: w285 -> [w288]
                                i -> [w287]
                                n875 = Not Equal?(x=w288, y=w287) -> (x != y?=w289:bool)
                                n876 = case shown="真" w289 {
                                tunnel: w287 -> [_ w290]
                                frame False {
                                }
                                frame True {
                                n877 = local read "数组_选择?"() -> (w294:bool[][])
                                n878 = Initialize Array(FALSE, 16 ("维数大小")) -> (w291:bool[])
                                n879 = Replace Array Subset(array=w294, new element=w291, index (row)=w290) -> (w295:bool[][])  [unwired: 1 in]
                                n880 = local write "数组_选择?"(w295) -> ()
                                }
                                }
                              }
                            }
                            frame #1 {
                            }
                          }
                        }
                      }
                      n881 = local write "保持输入"(w274) -> ()
                      n882 = property on="btn_开始试验" class="Bool"("DisabledEnum"=w275) -> ()  [unwired: 2 in, 2 out]
                    }
                  }
                }
              }
            }
          }
          frame #3 {
            n883 = local read "数组_选择?"() -> (w301:bool[][])
            n884 = Or Array Elements(Boolean array=w301) -> (logical OR=w300:bool)
            n885 = case shown="真" w300 {
              tunnel: w299 -> [_ w304]
              tunnel: w298 -> [_ w303]
              frame False {
                n886 = call "显示对话框信息"("Message"="请选择数字量输入路数") -> ()  [unwired: 9 in, 2 out]
              }
              frame True {
                n887 = Send Notification(notification="DInput" ("通知"), notifier=w304, error in (no error)=w303) -> ()  [unwired: 2 out]
              }
            }
          }
        }
      }
      event "保持输入": Value Change {
        n888 = event-data() -> ()  [unwired: 1 in, 5 out]
        n889 = property on="btn_开始试验" class="Bool"("DisabledEnum"=T1."Enabled" ("禁用")) -> ()  [unwired: 2 in, 2 out]
      }
      event "btn_全选": Value Change {
        w307 = TRUE ("单选_第41路")
        n890 = event-data() -> ()  [unwired: 1 in, 5 out]
        n891 = local write "单选_第1路"(w307) -> ()
        n892 = local write "单选_第2路"(w307) -> ()
        n893 = local write "单选_第3路"(w307) -> ()
        n894 = local write "单选_第4路"(w307) -> ()
        n895 = local write "单选_第5路"(w307) -> ()
        n896 = local write "单选_第6路"(w307) -> ()
        n897 = local write "单选_第7路"(w307) -> ()
        n898 = local write "单选_第8路"(w307) -> ()
        n899 = local write "单选_第9路"(w307) -> ()
        n900 = local write "单选_第10路"(w307) -> ()
        n901 = local write "单选_第11路"(w307) -> ()
        n902 = local write "单选_第12路"(w307) -> ()
        n903 = local write "单选_第13路"(w307) -> ()
        n904 = local write "单选_第14路"(w307) -> ()
        n905 = local write "单选_第15路"(w307) -> ()
        n906 = local write "单选_第16路"(w307) -> ()
        n907 = local write "单选_第17路"(w307) -> ()
        n908 = local write "单选_第18路"(w307) -> ()
        n909 = local write "单选_第19路"(w307) -> ()
        n910 = local write "单选_第20路"(w307) -> ()
        n911 = local write "单选_第21路"(w307) -> ()
        n912 = local write "单选_第22路"(w307) -> ()
        n913 = local write "单选_第23路"(w307) -> ()
        n914 = local write "单选_第24路"(w307) -> ()
        n915 = local write "单选_第25路"(w307) -> ()
        n916 = local write "单选_第26路"(w307) -> ()
        n917 = local write "单选_第27路"(w307) -> ()
        n918 = local write "单选_第28路"(w307) -> ()
        n919 = local write "单选_第29路"(w307) -> ()
        n920 = local write "单选_第30路"(w307) -> ()
        n921 = local write "单选_第31路"(w307) -> ()
        n922 = local write "单选_第32路"(w307) -> ()
        n923 = local write "单选_第33路"(w307) -> ()
        n924 = local write "单选_第34路"(w307) -> ()
        n925 = local write "单选_第35路"(w307) -> ()
        n926 = local write "单选_第36路"(w307) -> ()
        n927 = local write "单选_第37路"(w307) -> ()
        n928 = local write "单选_第38路"(w307) -> ()
        n929 = local write "单选_第39路"(w307) -> ()
        n930 = local write "单选_第40路"(w307) -> ()
        n931 = local write "单选_第41路"(w307) -> ()
        n932 = local write "单选_第42路"(w307) -> ()
        n933 = local write "单选_第43路"(w307) -> ()
        n934 = local write "单选_第44路"(w307) -> ()
        n935 = local write "单选_第45路"(w307) -> ()
        n936 = local write "单选_第46路"(w307) -> ()
        n937 = local write "单选_第47路"(w307) -> ()
        n938 = local write "单选_第48路"(w307) -> ()
        n939 = local write "单选_第49路"(w307) -> ()
        n940 = local write "单选_第50路"(w307) -> ()
        n941 = local write "单选_第51路"(w307) -> ()
        n942 = local write "单选_第52路"(w307) -> ()
        n943 = local write "单选_第53路"(w307) -> ()
        n944 = local write "单选_第54路"(w307) -> ()
        n945 = local write "单选_第55路"(w307) -> ()
        n946 = local write "单选_第56路"(w307) -> ()
        n947 = local write "单选_第57路"(w307) -> ()
        n948 = local write "单选_第58路"(w307) -> ()
        n949 = local write "单选_第59路"(w307) -> ()
        n950 = local write "单选_第60路"(w307) -> ()
        n951 = local write "单选_第61路"(w307) -> ()
        n952 = local write "单选_第62路"(w307) -> ()
        n953 = local write "单选_第63路"(w307) -> ()
        n954 = local write "单选_第64路"(w307) -> ()
        n955 = local write "单选_第71路"(w307) -> ()
        n956 = local write "单选_第79路"(w307) -> ()
        n957 = local write "单选_第65路"(w307) -> ()
        n958 = local write "单选_第66路"(w307) -> ()
        n959 = local write "单选_第67路"(w307) -> ()
        n960 = local write "单选_第68路"(w307) -> ()
        n961 = local write "单选_第69路"(w307) -> ()
        n962 = local write "单选_第70路"(w307) -> ()
        n963 = local write "单选_第72路"(w307) -> ()
        n964 = local write "单选_第73路"(w307) -> ()
        n965 = local write "单选_第74路"(w307) -> ()
        n966 = local write "单选_第75路"(w307) -> ()
        n967 = local write "单选_第76路"(w307) -> ()
        n968 = local write "单选_第77路"(w307) -> ()
        n969 = local write "单选_第78路"(w307) -> ()
        n970 = local write "单选_第80路"(w307) -> ()
      }
      event "btn_反选": Value Change {
        n971 = event-data() -> ()  [unwired: 1 in, 5 out]
        n972 = local read "单选_第1路"() -> (w467:bool)
        n973 = local read "单选_第2路"() -> (w465:bool)
        n974 = local read "单选_第3路"() -> (w463:bool)
        n975 = local read "单选_第4路"() -> (w461:bool)
        n976 = local read "单选_第5路"() -> (w459:bool)
        n977 = local read "单选_第6路"() -> (w457:bool)
        n978 = local read "单选_第7路"() -> (w456:bool)
        n979 = local read "单选_第8路"() -> (w455:bool)
        n980 = local read "单选_第9路"() -> (w454:bool)
        n981 = local read "单选_第10路"() -> (w453:bool)
        n982 = local read "单选_第11路"() -> (w452:bool)
        n983 = local read "单选_第12路"() -> (w451:bool)
        n984 = local read "单选_第13路"() -> (w450:bool)
        n985 = local read "单选_第14路"() -> (w449:bool)
        n986 = local read "单选_第15路"() -> (w448:bool)
        n987 = local read "单选_第16路"() -> (w447:bool)
        n988 = local read "单选_第17路"() -> (w446:bool)
        n989 = local read "单选_第18路"() -> (w445:bool)
        n990 = local read "单选_第19路"() -> (w444:bool)
        n991 = local read "单选_第20路"() -> (w443:bool)
        n992 = local read "单选_第21路"() -> (w442:bool)
        n993 = local read "单选_第22路"() -> (w441:bool)
        n994 = local read "单选_第23路"() -> (w440:bool)
        n995 = local read "单选_第24路"() -> (w439:bool)
        n996 = local read "单选_第25路"() -> (w438:bool)
        n997 = local read "单选_第26路"() -> (w437:bool)
        n998 = local read "单选_第27路"() -> (w436:bool)
        n999 = local read "单选_第28路"() -> (w435:bool)
        n1000 = local read "单选_第29路"() -> (w434:bool)
        n1001 = local read "单选_第30路"() -> (w433:bool)
        n1002 = local read "单选_第31路"() -> (w432:bool)
        n1003 = local read "单选_第32路"() -> (w431:bool)
        n1004 = local read "单选_第33路"() -> (w430:bool)
        n1005 = local read "单选_第34路"() -> (w429:bool)
        n1006 = local read "单选_第35路"() -> (w428:bool)
        n1007 = local read "单选_第36路"() -> (w427:bool)
        n1008 = local read "单选_第37路"() -> (w426:bool)
        n1009 = local read "单选_第38路"() -> (w425:bool)
        n1010 = local read "单选_第39路"() -> (w424:bool)
        n1011 = local read "单选_第40路"() -> (w423:bool)
        n1012 = Not(x=w467) -> (.not. x?=w466:bool)
        n1013 = Not(x=w465) -> (.not. x?=w464:bool)
        n1014 = Not(x=w463) -> (.not. x?=w462:bool)
        n1015 = Not(x=w461) -> (.not. x?=w460:bool)
        n1016 = Not(x=w459) -> (.not. x?=w458:bool)
        n1017 = Not(x=w457) -> (.not. x?=w422:bool)
        n1018 = Not(x=w456) -> (.not. x?=w421:bool)
        n1019 = Not(x=w455) -> (.not. x?=w420:bool)
        n1020 = Not(x=w454) -> (.not. x?=w419:bool)
        n1021 = Not(x=w453) -> (.not. x?=w418:bool)
        n1022 = Not(x=w452) -> (.not. x?=w417:bool)
        n1023 = Not(x=w451) -> (.not. x?=w416:bool)
        n1024 = Not(x=w450) -> (.not. x?=w415:bool)
        n1025 = Not(x=w449) -> (.not. x?=w414:bool)
        n1026 = Not(x=w448) -> (.not. x?=w413:bool)
        n1027 = Not(x=w447) -> (.not. x?=w412:bool)
        n1028 = Not(x=w446) -> (.not. x?=w411:bool)
        n1029 = Not(x=w445) -> (.not. x?=w410:bool)
        n1030 = Not(x=w444) -> (.not. x?=w409:bool)
        n1031 = Not(x=w443) -> (.not. x?=w408:bool)
        n1032 = Not(x=w442) -> (.not. x?=w407:bool)
        n1033 = Not(x=w441) -> (.not. x?=w406:bool)
        n1034 = Not(x=w440) -> (.not. x?=w405:bool)
        n1035 = Not(x=w439) -> (.not. x?=w404:bool)
        n1036 = Not(x=w438) -> (.not. x?=w403:bool)
        n1037 = Not(x=w437) -> (.not. x?=w402:bool)
        n1038 = Not(x=w436) -> (.not. x?=w401:bool)
        n1039 = Not(x=w435) -> (.not. x?=w400:bool)
        n1040 = Not(x=w434) -> (.not. x?=w399:bool)
        n1041 = Not(x=w433) -> (.not. x?=w398:bool)
        n1042 = Not(x=w432) -> (.not. x?=w397:bool)
        n1043 = Not(x=w431) -> (.not. x?=w396:bool)
        n1044 = Not(x=w430) -> (.not. x?=w395:bool)
        n1045 = Not(x=w429) -> (.not. x?=w394:bool)
        n1046 = Not(x=w428) -> (.not. x?=w393:bool)
        n1047 = Not(x=w427) -> (.not. x?=w392:bool)
        n1048 = Not(x=w426) -> (.not. x?=w391:bool)
        n1049 = Not(x=w425) -> (.not. x?=w390:bool)
        n1050 = Not(x=w424) -> (.not. x?=w389:bool)
        n1051 = Not(x=w423) -> (.not. x?=w388:bool)
        n1052 = local write "单选_第1路"(w466) -> ()
        n1053 = local write "单选_第2路"(w464) -> ()
        n1054 = local write "单选_第3路"(w462) -> ()
        n1055 = local write "单选_第4路"(w460) -> ()
        n1056 = local write "单选_第5路"(w458) -> ()
        n1057 = local write "单选_第6路"(w422) -> ()
        n1058 = local write "单选_第7路"(w421) -> ()
        n1059 = local write "单选_第8路"(w420) -> ()
        n1060 = local write "单选_第9路"(w419) -> ()
        n1061 = local write "单选_第10路"(w418) -> ()
        n1062 = local write "单选_第11路"(w417) -> ()
        n1063 = local write "单选_第12路"(w416) -> ()
        n1064 = local write "单选_第13路"(w415) -> ()
        n1065 = local write "单选_第14路"(w414) -> ()
        n1066 = local write "单选_第15路"(w413) -> ()
        n1067 = local write "单选_第16路"(w412) -> ()
        n1068 = local write "单选_第17路"(w411) -> ()
        n1069 = local write "单选_第18路"(w410) -> ()
        n1070 = local write "单选_第19路"(w409) -> ()
        n1071 = local write "单选_第20路"(w408) -> ()
        n1072 = local write "单选_第21路"(w407) -> ()
        n1073 = local write "单选_第22路"(w406) -> ()
        n1074 = local write "单选_第23路"(w405) -> ()
        n1075 = local write "单选_第24路"(w404) -> ()
        n1076 = local write "单选_第25路"(w403) -> ()
        n1077 = local write "单选_第26路"(w402) -> ()
        n1078 = local write "单选_第27路"(w401) -> ()
        n1079 = local write "单选_第28路"(w400) -> ()
        n1080 = local write "单选_第29路"(w399) -> ()
        n1081 = local write "单选_第30路"(w398) -> ()
        n1082 = local write "单选_第31路"(w397) -> ()
        n1083 = local write "单选_第32路"(w396) -> ()
        n1084 = local write "单选_第33路"(w395) -> ()
        n1085 = local write "单选_第34路"(w394) -> ()
        n1086 = local write "单选_第35路"(w393) -> ()
        n1087 = local write "单选_第36路"(w392) -> ()
        n1088 = local write "单选_第37路"(w391) -> ()
        n1089 = local write "单选_第38路"(w390) -> ()
        n1090 = local write "单选_第39路"(w389) -> ()
        n1091 = local write "单选_第40路"(w388) -> ()
        n1092 = local read "单选_第71路"() -> (w357:bool)
        n1093 = local read "单选_第79路"() -> (w349:bool)
        n1094 = local read "单选_第41路"() -> (w387:bool)
        n1095 = local read "单选_第42路"() -> (w386:bool)
        n1096 = local read "单选_第43路"() -> (w385:bool)
        n1097 = local read "单选_第44路"() -> (w384:bool)
        n1098 = local read "单选_第45路"() -> (w383:bool)
        n1099 = local read "单选_第46路"() -> (w382:bool)
        n1100 = local read "单选_第47路"() -> (w381:bool)
        n1101 = local read "单选_第48路"() -> (w380:bool)
        n1102 = local read "单选_第49路"() -> (w379:bool)
        n1103 = local read "单选_第50路"() -> (w378:bool)
        n1104 = local read "单选_第51路"() -> (w377:bool)
        n1105 = local read "单选_第52路"() -> (w376:bool)
        n1106 = local read "单选_第53路"() -> (w375:bool)
        n1107 = local read "单选_第54路"() -> (w374:bool)
        n1108 = local read "单选_第55路"() -> (w373:bool)
        n1109 = local read "单选_第56路"() -> (w372:bool)
        n1110 = local read "单选_第57路"() -> (w371:bool)
        n1111 = local read "单选_第58路"() -> (w370:bool)
        n1112 = local read "单选_第59路"() -> (w369:bool)
        n1113 = local read "单选_第60路"() -> (w368:bool)
        n1114 = local read "单选_第61路"() -> (w367:bool)
        n1115 = local read "单选_第62路"() -> (w366:bool)
        n1116 = local read "单选_第63路"() -> (w365:bool)
        n1117 = local read "单选_第64路"() -> (w364:bool)
        n1118 = local read "单选_第65路"() -> (w363:bool)
        n1119 = local read "单选_第66路"() -> (w362:bool)
        n1120 = local read "单选_第67路"() -> (w361:bool)
        n1121 = local read "单选_第68路"() -> (w360:bool)
        n1122 = local read "单选_第69路"() -> (w359:bool)
        n1123 = local read "单选_第70路"() -> (w358:bool)
        n1124 = local read "单选_第72路"() -> (w356:bool)
        n1125 = local read "单选_第73路"() -> (w355:bool)
        n1126 = local read "单选_第74路"() -> (w354:bool)
        n1127 = local read "单选_第75路"() -> (w353:bool)
        n1128 = local read "单选_第76路"() -> (w352:bool)
        n1129 = local read "单选_第77路"() -> (w351:bool)
        n1130 = local read "单选_第78路"() -> (w350:bool)
        n1131 = local read "单选_第80路"() -> (w348:bool)
        n1132 = Not(x=w387) -> (.not. x?=w347:bool)
        n1133 = Not(x=w386) -> (.not. x?=w346:bool)
        n1134 = Not(x=w385) -> (.not. x?=w345:bool)
        n1135 = Not(x=w384) -> (.not. x?=w344:bool)
        n1136 = Not(x=w383) -> (.not. x?=w343:bool)
        n1137 = Not(x=w382) -> (.not. x?=w342:bool)
        n1138 = Not(x=w381) -> (.not. x?=w341:bool)
        n1139 = Not(x=w380) -> (.not. x?=w340:bool)
        n1140 = Not(x=w379) -> (.not. x?=w339:bool)
        n1141 = Not(x=w378) -> (.not. x?=w338:bool)
        n1142 = Not(x=w377) -> (.not. x?=w337:bool)
        n1143 = Not(x=w376) -> (.not. x?=w336:bool)
        n1144 = Not(x=w375) -> (.not. x?=w335:bool)
        n1145 = Not(x=w374) -> (.not. x?=w334:bool)
        n1146 = Not(x=w373) -> (.not. x?=w333:bool)
        n1147 = Not(x=w372) -> (.not. x?=w332:bool)
        n1148 = Not(x=w371) -> (.not. x?=w331:bool)
        n1149 = Not(x=w370) -> (.not. x?=w330:bool)
        n1150 = Not(x=w369) -> (.not. x?=w329:bool)
        n1151 = Not(x=w368) -> (.not. x?=w328:bool)
        n1152 = Not(x=w367) -> (.not. x?=w327:bool)
        n1153 = Not(x=w366) -> (.not. x?=w326:bool)
        n1154 = Not(x=w365) -> (.not. x?=w325:bool)
        n1155 = Not(x=w364) -> (.not. x?=w324:bool)
        n1156 = Not(x=w363) -> (.not. x?=w323:bool)
        n1157 = Not(x=w362) -> (.not. x?=w322:bool)
        n1158 = Not(x=w361) -> (.not. x?=w321:bool)
        n1159 = Not(x=w360) -> (.not. x?=w320:bool)
        n1160 = Not(x=w359) -> (.not. x?=w319:bool)
        n1161 = Not(x=w358) -> (.not. x?=w318:bool)
        n1162 = Not(x=w357) -> (.not. x?=w317:bool)
        n1163 = Not(x=w356) -> (.not. x?=w316:bool)
        n1164 = Not(x=w355) -> (.not. x?=w315:bool)
        n1165 = Not(x=w354) -> (.not. x?=w314:bool)
        n1166 = Not(x=w353) -> (.not. x?=w313:bool)
        n1167 = Not(x=w352) -> (.not. x?=w312:bool)
        n1168 = Not(x=w351) -> (.not. x?=w311:bool)
        n1169 = Not(x=w350) -> (.not. x?=w310:bool)
        n1170 = Not(x=w349) -> (.not. x?=w309:bool)
        n1171 = Not(x=w348) -> (.not. x?=w308:bool)
        n1172 = local write "单选_第71路"(w317) -> ()
        n1173 = local write "单选_第79路"(w309) -> ()
        n1174 = local write "单选_第41路"(w347) -> ()
        n1175 = local write "单选_第42路"(w346) -> ()
        n1176 = local write "单选_第43路"(w345) -> ()
        n1177 = local write "单选_第44路"(w344) -> ()
        n1178 = local write "单选_第45路"(w343) -> ()
        n1179 = local write "单选_第46路"(w342) -> ()
        n1180 = local write "单选_第47路"(w341) -> ()
        n1181 = local write "单选_第48路"(w340) -> ()
        n1182 = local write "单选_第49路"(w339) -> ()
        n1183 = local write "单选_第50路"(w338) -> ()
        n1184 = local write "单选_第51路"(w337) -> ()
        n1185 = local write "单选_第52路"(w336) -> ()
        n1186 = local write "单选_第53路"(w335) -> ()
        n1187 = local write "单选_第54路"(w334) -> ()
        n1188 = local write "单选_第55路"(w333) -> ()
        n1189 = local write "单选_第56路"(w332) -> ()
        n1190 = local write "单选_第57路"(w331) -> ()
        n1191 = local write "单选_第58路"(w330) -> ()
        n1192 = local write "单选_第59路"(w329) -> ()
        n1193 = local write "单选_第60路"(w328) -> ()
        n1194 = local write "单选_第61路"(w327) -> ()
        n1195 = local write "单选_第62路"(w326) -> ()
        n1196 = local write "单选_第63路"(w325) -> ()
        n1197 = local write "单选_第64路"(w324) -> ()
        n1198 = local write "单选_第65路"(w323) -> ()
        n1199 = local write "单选_第66路"(w322) -> ()
        n1200 = local write "单选_第67路"(w321) -> ()
        n1201 = local write "单选_第68路"(w320) -> ()
        n1202 = local write "单选_第69路"(w319) -> ()
        n1203 = local write "单选_第70路"(w318) -> ()
        n1204 = local write "单选_第72路"(w316) -> ()
        n1205 = local write "单选_第73路"(w315) -> ()
        n1206 = local write "单选_第74路"(w314) -> ()
        n1207 = local write "单选_第75路"(w313) -> ()
        n1208 = local write "单选_第76路"(w312) -> ()
        n1209 = local write "单选_第77路"(w311) -> ()
        n1210 = local write "单选_第78路"(w310) -> ()
        n1211 = local write "单选_第80路"(w308) -> ()
      }
      event "btn_置1": Value Change {
        w468 = enum16{"0", "1"}."1" ("输入值_41")
        n1212 = event-data() -> ()  [unwired: 1 in, 5 out]
        n1213 = local write "输入值_1"(w468) -> ()
        n1214 = local write "输入值_2"(w468) -> ()
        n1215 = local write "输入值_3"(w468) -> ()
        n1216 = local write "输入值_4"(w468) -> ()
        n1217 = local write "输入值_5"(w468) -> ()
        n1218 = local write "输入值_6"(w468) -> ()
        n1219 = local write "输入值_7"(w468) -> ()
        n1220 = local write "输入值_8"(w468) -> ()
        n1221 = local write "输入值_9"(w468) -> ()
        n1222 = local write "输入值_10"(w468) -> ()
        n1223 = local write "输入值_11"(w468) -> ()
        n1224 = local write "输入值_12"(w468) -> ()
        n1225 = local write "输入值_13"(w468) -> ()
        n1226 = local write "输入值_14"(w468) -> ()
        n1227 = local write "输入值_15"(w468) -> ()
        n1228 = local write "输入值_16"(w468) -> ()
        n1229 = local write "输入值_17"(w468) -> ()
        n1230 = local write "输入值_18"(w468) -> ()
        n1231 = local write "输入值_19"(w468) -> ()
        n1232 = local write "输入值_20"(w468) -> ()
        n1233 = local write "输入值_21"(w468) -> ()
        n1234 = local write "输入值_22"(w468) -> ()
        n1235 = local write "输入值_23"(w468) -> ()
        n1236 = local write "输入值_24"(w468) -> ()
        n1237 = local write "输入值_25"(w468) -> ()
        n1238 = local write "输入值_26"(w468) -> ()
        n1239 = local write "输入值_27"(w468) -> ()
        n1240 = local write "输入值_28"(w468) -> ()
        n1241 = local write "输入值_29"(w468) -> ()
        n1242 = local write "输入值_30"(w468) -> ()
        n1243 = local write "输入值_31"(w468) -> ()
        n1244 = local write "输入值_32"(w468) -> ()
        n1245 = local write "输入值_33"(w468) -> ()
        n1246 = local write "输入值_34"(w468) -> ()
        n1247 = local write "输入值_35"(w468) -> ()
        n1248 = local write "输入值_36"(w468) -> ()
        n1249 = local write "输入值_37"(w468) -> ()
        n1250 = local write "输入值_38"(w468) -> ()
        n1251 = local write "输入值_39"(w468) -> ()
        n1252 = local write "输入值_40"(w468) -> ()
        n1253 = local write "输入值_41"(w468) -> ()
        n1254 = local write "输入值_42"(w468) -> ()
        n1255 = local write "输入值_43"(w468) -> ()
        n1256 = local write "输入值_44"(w468) -> ()
        n1257 = local write "输入值_45"(w468) -> ()
        n1258 = local write "输入值_46"(w468) -> ()
        n1259 = local write "输入值_47"(w468) -> ()
        n1260 = local write "输入值_48"(w468) -> ()
        n1261 = local write "输入值_49"(w468) -> ()
        n1262 = local write "输入值_50"(w468) -> ()
        n1263 = local write "输入值_51"(w468) -> ()
        n1264 = local write "输入值_52"(w468) -> ()
        n1265 = local write "输入值_53"(w468) -> ()
        n1266 = local write "输入值_54"(w468) -> ()
        n1267 = local write "输入值_55"(w468) -> ()
        n1268 = local write "输入值_56"(w468) -> ()
        n1269 = local write "输入值_57"(w468) -> ()
        n1270 = local write "输入值_58"(w468) -> ()
        n1271 = local write "输入值_59"(w468) -> ()
        n1272 = local write "输入值_60"(w468) -> ()
        n1273 = local write "输入值_61"(w468) -> ()
        n1274 = local write "输入值_62"(w468) -> ()
        n1275 = local write "输入值_63"(w468) -> ()
        n1276 = local write "输入值_64"(w468) -> ()
        n1277 = local write "输入值_65"(w468) -> ()
        n1278 = local write "输入值_66"(w468) -> ()
        n1279 = local write "输入值_67"(w468) -> ()
        n1280 = local write "输入值_68"(w468) -> ()
        n1281 = local write "输入值_69"(w468) -> ()
        n1282 = local write "输入值_70"(w468) -> ()
        n1283 = local write "输入值_71"(w468) -> ()
        n1284 = local write "输入值_72"(w468) -> ()
        n1285 = local write "输入值_73"(w468) -> ()
        n1286 = local write "输入值_74"(w468) -> ()
        n1287 = local write "输入值_75"(w468) -> ()
        n1288 = local write "输入值_76"(w468) -> ()
        n1289 = local write "输入值_77"(w468) -> ()
        n1290 = local write "输入值_78"(w468) -> ()
        n1291 = local write "输入值_79"(w468) -> ()
        n1292 = local write "输入值_80"(w468) -> ()
      }
      event "btn_置0": Value Change {
        w469 = enum16{"0", "1"}."0" ("输入值_41")
        n1293 = event-data() -> ()  [unwired: 1 in, 5 out]
        n1294 = local write "输入值_1"(w469) -> ()
        n1295 = local write "输入值_2"(w469) -> ()
        n1296 = local write "输入值_3"(w469) -> ()
        n1297 = local write "输入值_4"(w469) -> ()
        n1298 = local write "输入值_5"(w469) -> ()
        n1299 = local write "输入值_6"(w469) -> ()
        n1300 = local write "输入值_7"(w469) -> ()
        n1301 = local write "输入值_8"(w469) -> ()
        n1302 = local write "输入值_9"(w469) -> ()
        n1303 = local write "输入值_10"(w469) -> ()
        n1304 = local write "输入值_11"(w469) -> ()
        n1305 = local write "输入值_12"(w469) -> ()
        n1306 = local write "输入值_13"(w469) -> ()
        n1307 = local write "输入值_14"(w469) -> ()
        n1308 = local write "输入值_15"(w469) -> ()
        n1309 = local write "输入值_16"(w469) -> ()
        n1310 = local write "输入值_17"(w469) -> ()
        n1311 = local write "输入值_18"(w469) -> ()
        n1312 = local write "输入值_19"(w469) -> ()
        n1313 = local write "输入值_20"(w469) -> ()
        n1314 = local write "输入值_21"(w469) -> ()
        n1315 = local write "输入值_22"(w469) -> ()
        n1316 = local write "输入值_23"(w469) -> ()
        n1317 = local write "输入值_24"(w469) -> ()
        n1318 = local write "输入值_25"(w469) -> ()
        n1319 = local write "输入值_26"(w469) -> ()
        n1320 = local write "输入值_27"(w469) -> ()
        n1321 = local write "输入值_28"(w469) -> ()
        n1322 = local write "输入值_29"(w469) -> ()
        n1323 = local write "输入值_30"(w469) -> ()
        n1324 = local write "输入值_31"(w469) -> ()
        n1325 = local write "输入值_32"(w469) -> ()
        n1326 = local write "输入值_33"(w469) -> ()
        n1327 = local write "输入值_34"(w469) -> ()
        n1328 = local write "输入值_35"(w469) -> ()
        n1329 = local write "输入值_36"(w469) -> ()
        n1330 = local write "输入值_37"(w469) -> ()
        n1331 = local write "输入值_38"(w469) -> ()
        n1332 = local write "输入值_39"(w469) -> ()
        n1333 = local write "输入值_40"(w469) -> ()
        n1334 = local write "输入值_41"(w469) -> ()
        n1335 = local write "输入值_42"(w469) -> ()
        n1336 = local write "输入值_43"(w469) -> ()
        n1337 = local write "输入值_44"(w469) -> ()
        n1338 = local write "输入值_45"(w469) -> ()
        n1339 = local write "输入值_46"(w469) -> ()
        n1340 = local write "输入值_47"(w469) -> ()
        n1341 = local write "输入值_48"(w469) -> ()
        n1342 = local write "输入值_49"(w469) -> ()
        n1343 = local write "输入值_50"(w469) -> ()
        n1344 = local write "输入值_51"(w469) -> ()
        n1345 = local write "输入值_52"(w469) -> ()
        n1346 = local write "输入值_53"(w469) -> ()
        n1347 = local write "输入值_54"(w469) -> ()
        n1348 = local write "输入值_55"(w469) -> ()
        n1349 = local write "输入值_56"(w469) -> ()
        n1350 = local write "输入值_57"(w469) -> ()
        n1351 = local write "输入值_58"(w469) -> ()
        n1352 = local write "输入值_59"(w469) -> ()
        n1353 = local write "输入值_60"(w469) -> ()
        n1354 = local write "输入值_61"(w469) -> ()
        n1355 = local write "输入值_62"(w469) -> ()
        n1356 = local write "输入值_63"(w469) -> ()
        n1357 = local write "输入值_64"(w469) -> ()
        n1358 = local write "输入值_65"(w469) -> ()
        n1359 = local write "输入值_66"(w469) -> ()
        n1360 = local write "输入值_67"(w469) -> ()
        n1361 = local write "输入值_68"(w469) -> ()
        n1362 = local write "输入值_69"(w469) -> ()
        n1363 = local write "输入值_70"(w469) -> ()
        n1364 = local write "输入值_71"(w469) -> ()
        n1365 = local write "输入值_72"(w469) -> ()
        n1366 = local write "输入值_73"(w469) -> ()
        n1367 = local write "输入值_74"(w469) -> ()
        n1368 = local write "输入值_75"(w469) -> ()
        n1369 = local write "输入值_76"(w469) -> ()
        n1370 = local write "输入值_77"(w469) -> ()
        n1371 = local write "输入值_78"(w469) -> ()
        n1372 = local write "输入值_79"(w469) -> ()
        n1373 = local write "输入值_80"(w469) -> ()
      }
    }
  }
  n1374 = stacked-sequence {
    frame #0 {
      w473 = T1."Enabled" ("禁用")
      w474 = cluster{u32, u32}[] [{9868950, 9868950}]
      w475 = 0 ("同步_A2")
      w491 = T1."Disabled" ("禁用")
      n1375 = property on="测试结论" class="Str"("Text.TextColor"=u32 0) -> ()  [unwired: 2 in, 2 out]
      n1376 = local write "测试结论"("") -> ()
      n1377 = property on="D_IN_1" class="Tbl (严格)"("DisabledEnum"=w491) -> ()  [unwired: 2 in, 2 out]
      n1378 = property on="D_IN_2" class="Tbl (严格)"("DisabledEnum"=w491) -> ()  [unwired: 2 in, 2 out]
      n1379 = property on="D_IN_3" class="Tbl (严格)"("DisabledEnum"=w491) -> ()  [unwired: 2 in, 2 out]
      n1380 = property on="D_IN_4" class="Tbl (严格)"("DisabledEnum"=w491) -> ()  [unwired: 2 in, 2 out]
      n1381 = property on="D_IN_5" class="Tbl (严格)"("DisabledEnum"=w491) -> ()  [unwired: 2 in, 2 out]
      n1382 = property on="light_1" class="Bool (严格)"("Colors [4]"=w474) -> ()  [unwired: 2 in, 2 out]
      n1383 = property on="light_2" class="Bool (严格)"("Colors [4]"=w474) -> ()  [unwired: 2 in, 2 out]
      n1384 = property on="light_3" class="Bool (严格)"("Colors [4]"=w474) -> ()  [unwired: 2 in, 2 out]
      n1385 = property on="light_4" class="Bool (严格)"("Colors [4]"=w474) -> ()  [unwired: 2 in, 2 out]
      n1386 = property on="light_5" class="Bool (严格)"("Colors [4]"=w474) -> ()  [unwired: 2 in, 2 out]
      n1387 = property on="light_6" class="Bool (严格)"("Colors [4]"=w474) -> ()  [unwired: 2 in, 2 out]
      n1388 = property on="light_7" class="Bool (严格)"("Colors [4]"=w474) -> ()  [unwired: 2 in, 2 out]
      n1389 = property on="light_8" class="Bool (严格)"("Colors [4]"=w474) -> ()  [unwired: 2 in, 2 out]
      n1390 = property on="light_9" class="Bool (严格)"("Colors [4]"=w474) -> ()  [unwired: 2 in, 2 out]
      n1391 = property on="light_10" class="Bool (严格)"("Colors [4]"=w474) -> ()  [unwired: 2 in, 2 out]
      n1392 = property on="light_11" class="Bool (严格)"("Colors [4]"=w474) -> ()  [unwired: 2 in, 2 out]
      n1393 = property on="light_12" class="Bool (严格)"("Colors [4]"=w474) -> ()  [unwired: 2 in, 2 out]
      n1394 = property on="light_13" class="Bool (严格)"("Colors [4]"=w474) -> ()  [unwired: 2 in, 2 out]
      n1395 = property on="light_14" class="Bool (严格)"("Colors [4]"=w474) -> ()  [unwired: 2 in, 2 out]
      n1396 = property on="light_15" class="Bool (严格)"("Colors [4]"=w474) -> ()  [unwired: 2 in, 2 out]
      n1397 = property on="light_16" class="Bool (严格)"("Colors [4]"=w474) -> ()  [unwired: 2 in, 2 out]
      n1398 = property on="light_17" class="Bool (严格)"("Colors [4]"=w474) -> ()  [unwired: 2 in, 2 out]
      n1399 = property on="light_18" class="Bool (严格)"("Colors [4]"=w474) -> ()  [unwired: 2 in, 2 out]
      n1400 = property on="light_19" class="Bool (严格)"("Colors [4]"=w474) -> ()  [unwired: 2 in, 2 out]
      n1401 = property on="light_20" class="Bool (严格)"("Colors [4]"=w474) -> ()  [unwired: 2 in, 2 out]
      n1402 = property on="light_21" class="Bool (严格)"("Colors [4]"=w474) -> ()  [unwired: 2 in, 2 out]
      n1403 = property on="light_22" class="Bool (严格)"("Colors [4]"=w474) -> ()  [unwired: 2 in, 2 out]
      n1404 = property on="light_23" class="Bool (严格)"("Colors [4]"=w474) -> ()  [unwired: 2 in, 2 out]
      n1405 = property on="light_24" class="Bool (严格)"("Colors [4]"=w474) -> ()  [unwired: 2 in, 2 out]
      n1406 = property on="light_25" class="Bool (严格)"("Colors [4]"=w474) -> ()  [unwired: 2 in, 2 out]
      n1407 = property on="light_26" class="Bool (严格)"("Colors [4]"=w474) -> ()  [unwired: 2 in, 2 out]
      n1408 = property on="light_27" class="Bool (严格)"("Colors [4]"=w474) -> ()  [unwired: 2 in, 2 out]
      n1409 = property on="light_28" class="Bool (严格)"("Colors [4]"=w474) -> ()  [unwired: 2 in, 2 out]
      n1410 = property on="light_29" class="Bool (严格)"("Colors [4]"=w474) -> ()  [unwired: 2 in, 2 out]
      n1411 = property on="light_30" class="Bool (严格)"("Colors [4]"=w474) -> ()  [unwired: 2 in, 2 out]
      n1412 = property on="light_31" class="Bool (严格)"("Colors [4]"=w474) -> ()  [unwired: 2 in, 2 out]
      n1413 = property on="light_32" class="Bool (严格)"("Colors [4]"=w474) -> ()  [unwired: 2 in, 2 out]
      n1414 = property on="light_33" class="Bool (严格)"("Colors [4]"=w474) -> ()  [unwired: 2 in, 2 out]
      n1415 = property on="light_34" class="Bool (严格)"("Colors [4]"=w474) -> ()  [unwired: 2 in, 2 out]
      n1416 = property on="light_35" class="Bool (严格)"("Colors [4]"=w474) -> ()  [unwired: 2 in, 2 out]
      n1417 = property on="light_36" class="Bool (严格)"("Colors [4]"=w474) -> ()  [unwired: 2 in, 2 out]
      n1418 = property on="light_37" class="Bool (严格)"("Colors [4]"=w474) -> ()  [unwired: 2 in, 2 out]
      n1419 = property on="light_38" class="Bool (严格)"("Colors [4]"=w474) -> ()  [unwired: 2 in, 2 out]
      n1420 = property on="light_39" class="Bool (严格)"("Colors [4]"=w474) -> ()  [unwired: 2 in, 2 out]
      n1421 = property on="light_40" class="Bool (严格)"("Colors [4]"=w474) -> ()  [unwired: 2 in, 2 out]
      n1422 = property on="light_41" class="Bool (严格)"("Colors [4]"=w474) -> ()  [unwired: 2 in, 2 out]
      n1423 = property on="light_42" class="Bool (严格)"("Colors [4]"=w474) -> ()  [unwired: 2 in, 2 out]
      n1424 = property on="light_43" class="Bool (严格)"("Colors [4]"=w474) -> ()  [unwired: 2 in, 2 out]
      n1425 = property on="light_44" class="Bool (严格)"("Colors [4]"=w474) -> ()  [unwired: 2 in, 2 out]
      n1426 = property on="light_45" class="Bool (严格)"("Colors [4]"=w474) -> ()  [unwired: 2 in, 2 out]
      n1427 = property on="light_46" class="Bool (严格)"("Colors [4]"=w474) -> ()  [unwired: 2 in, 2 out]
      n1428 = property on="light_47" class="Bool (严格)"("Colors [4]"=w474) -> ()  [unwired: 2 in, 2 out]
      n1429 = property on="light_48" class="Bool (严格)"("Colors [4]"=w474) -> ()  [unwired: 2 in, 2 out]
      n1430 = property on="light_49" class="Bool (严格)"("Colors [4]"=w474) -> ()  [unwired: 2 in, 2 out]
      n1431 = property on="light_50" class="Bool (严格)"("Colors [4]"=w474) -> ()  [unwired: 2 in, 2 out]
      n1432 = property on="light_51" class="Bool (严格)"("Colors [4]"=w474) -> ()  [unwired: 2 in, 2 out]
      n1433 = property on="light_52" class="Bool (严格)"("Colors [4]"=w474) -> ()  [unwired: 2 in, 2 out]
      n1434 = property on="light_53" class="Bool (严格)"("Colors [4]"=w474) -> ()  [unwired: 2 in, 2 out]
      n1435 = property on="light_54" class="Bool (严格)"("Colors [4]"=w474) -> ()  [unwired: 2 in, 2 out]
      n1436 = property on="light_55" class="Bool (严格)"("Colors [4]"=w474) -> ()  [unwired: 2 in, 2 out]
      n1437 = property on="light_56" class="Bool (严格)"("Colors [4]"=w474) -> ()  [unwired: 2 in, 2 out]
      n1438 = property on="light_57" class="Bool (严格)"("Colors [4]"=w474) -> ()  [unwired: 2 in, 2 out]
      n1439 = property on="light_58" class="Bool (严格)"("Colors [4]"=w474) -> ()  [unwired: 2 in, 2 out]
      n1440 = property on="light_59" class="Bool (严格)"("Colors [4]"=w474) -> ()  [unwired: 2 in, 2 out]
      n1441 = property on="light_60" class="Bool (严格)"("Colors [4]"=w474) -> ()  [unwired: 2 in, 2 out]
      n1442 = property on="light_61" class="Bool (严格)"("Colors [4]"=w474) -> ()  [unwired: 2 in, 2 out]
      n1443 = property on="light_62" class="Bool (严格)"("Colors [4]"=w474) -> ()  [unwired: 2 in, 2 out]
      n1444 = property on="light_63" class="Bool (严格)"("Colors [4]"=w474) -> ()  [unwired: 2 in, 2 out]
      n1445 = property on="light_64" class="Bool (严格)"("Colors [4]"=w474) -> ()  [unwired: 2 in, 2 out]
      n1446 = property on="light_65" class="Bool (严格)"("Colors [4]"=w474) -> ()  [unwired: 2 in, 2 out]
      n1447 = property on="light_66" class="Bool (严格)"("Colors [4]"=w474) -> ()  [unwired: 2 in, 2 out]
      n1448 = property on="light_67" class="Bool (严格)"("Colors [4]"=w474) -> ()  [unwired: 2 in, 2 out]
      n1449 = property on="light_68" class="Bool (严格)"("Colors [4]"=w474) -> ()  [unwired: 2 in, 2 out]
      n1450 = property on="light_69" class="Bool (严格)"("Colors [4]"=w474) -> ()  [unwired: 2 in, 2 out]
      n1451 = property on="light_70" class="Bool (严格)"("Colors [4]"=w474) -> ()  [unwired: 2 in, 2 out]
      n1452 = property on="light_71" class="Bool (严格)"("Colors [4]"=w474) -> ()  [unwired: 2 in, 2 out]
      n1453 = property on="light_72" class="Bool (严格)"("Colors [4]"=w474) -> ()  [unwired: 2 in, 2 out]
      n1454 = property on="light_73" class="Bool (严格)"("Colors [4]"=w474) -> ()  [unwired: 2 in, 2 out]
      n1455 = property on="light_74" class="Bool (严格)"("Colors [4]"=w474) -> ()  [unwired: 2 in, 2 out]
      n1456 = property on="light_75" class="Bool (严格)"("Colors [4]"=w474) -> ()  [unwired: 2 in, 2 out]
      n1457 = property on="light_76" class="Bool (严格)"("Colors [4]"=w474) -> ()  [unwired: 2 in, 2 out]
      n1458 = property on="light_77" class="Bool (严格)"("Colors [4]"=w474) -> ()  [unwired: 2 in, 2 out]
      n1459 = property on="light_78" class="Bool (严格)"("Colors [4]"=w474) -> ()  [unwired: 2 in, 2 out]
      n1460 = property on="light_79" class="Bool (严格)"("Colors [4]"=w474) -> ()  [unwired: 2 in, 2 out]
      n1461 = property on="light_80" class="Bool (严格)"("Colors [4]"=w474) -> ()  [unwired: 2 in, 2 out]
      n1462 = local write "CAN端口"(u16 1 ("CAN端口")) -> ()
      n1463 = local write "关闭？"(FALSE) -> ()
      n1464 = for {
        N: 16 -> [_]
        i -> [w495]
        n1465 = for {
          N: 4 -> [_]
          tunnel: w495 -> [w499]
          i -> [w500]
          w497 = u32 24 ("活动单元格:单元格大小:高度")
          n1466 = Bundle(w499, w500) -> (w498:cluster{i32, i32})  [unwired: 1 in]
          n1467 = property on="D_IN_1" class="Tbl (严格)"("Active Cell"=w498) -> (error out=w501:errorcluster)  [unwired: 2 in, 1 out]
          n1468 = property on="D_IN_2" class="Tbl (严格)"("Active Cell"=w498) -> ()  [unwired: 2 in, 2 out]
          n1469 = property on="D_IN_3" class="Tbl (严格)"("Active Cell"=w498) -> ()  [unwired: 2 in, 2 out]
          n1470 = property on="D_IN_4" class="Tbl (严格)"("Active Cell"=w498) -> ()  [unwired: 2 in, 2 out]
          n1471 = property on="D_IN_5" class="Tbl (严格)"("Active Cell"=w498) -> ()  [unwired: 2 in, 2 out]
          n1472 = property on="D_IN_1" class="Tbl (严格)"(error in=w501, "Height"=w497) -> ()  [unwired: 1 in, 2 out]
          n1473 = property on="D_IN_2" class="Tbl (严格)"("Height"=w497) -> ()  [unwired: 2 in, 2 out]
          n1474 = property on="D_IN_3" class="Tbl (严格)"("Height"=w497) -> ()  [unwired: 2 in, 2 out]
          n1475 = property on="D_IN_4" class="Tbl (严格)"("Height"=w497) -> ()  [unwired: 2 in, 2 out]
          n1476 = property on="D_IN_5" class="Tbl (严格)"("Height"=w497) -> ()  [unwired: 2 in, 2 out]
        }
        n1477 = Wait Until Next ms Multiple(millisecond multiple=u32 10 ("毫秒倍数")) -> ()  [unwired: 1 out]
      }
      n1478 = Initialize Array("", 16 ("维数大小"), 4 ("维数大小")) -> (w485:string[][])
      n1479 = property on="btn_开始试验" class="Bool"("DisabledEnum"=w473) -> ()  [unwired: 2 in, 2 out]
      n1480 = property on="保持输入" class="Bool (严格)"("DisabledEnum"=w473) -> ()  [unwired: 2 in, 2 out]
      n1481 = local write "D_IN_1"(w485) -> ()
      n1482 = local write "D_IN_2"(w485) -> ()
      n1483 = local write "D_IN_3"(w485) -> ()
      n1484 = local write "D_IN_4"(w485) -> ()
      n1485 = local write "D_IN_5"(w485) -> ()
      n1486 = local write "同步_A2"(w475) -> ()
      n1487 = local write "同步_A1"(w475) -> ()
      n1488 = Initialize Array(FALSE, 6 ("维数大小"), 16 ("维数大小")) -> (w483:bool[][])
      n1489 = Initialize Array(enum16{"0", "1"}."0" ("输入值_32"), 6 ("维数大小"), 16 ("维数大小")) -> (w478:enum16{"0", "1"}[][])
      n1490 = local write "数组_选择?"(w483) -> ()
      n1491 = Initialize Array(u16 0, 6 ("维数大小")) -> (w472:u16[])
      n1492 = local write "数组_输入值"(w478) -> ()
      n1493 = local write "数组"(w472) -> ()
    }
  }
  n1494 = Obtain Notifier(name (unnamed)=w11, notification data type=w11) -> (notifier out=w15:refnum<notifier>, error out=w14:errorcluster)  [unwired: 2 in, 1 out]
  n1495 = disable-structure shown="禁用" {
    frame Disabled {
      n1496 = for {
        N: 40 -> [_]
        i -> [w504]
        n1497 = for {
          N: 4 -> [_]
          tunnel: w504 -> [w512]
          i -> [w509]
          n1498 = Bundle(w512, w509) -> (w508:cluster{i32, i32})  [unwired: 1 in]
          n1499 = Quotient & Remainder(x=w512, y=2) -> (x-y*floor(x/y)=w510:i32)  [unwired: 1 out]
          n1500 = property on="D_IN_1" class="Tbl (严格)"("Active Cell"=w508) -> (error out=w506:errorcluster)  [unwired: 2 in, 1 out]
          n1501 = Equal To 0?(x=w510) -> (x = 0?=w513:bool)
          n1502 = case shown="真" w513 {
            tunnel: [u32 16448250 u32 15723488] -> w507
            frame False {
            }
            frame True {
            }
          }
          n1503 = property on="D_IN_1" class="Tbl (严格)"(error in=w506, "Cell BG Color"=w507) -> ()  [unwired: 1 in, 2 out]
        }
        n1504 = Wait Until Next ms Multiple(millisecond multiple=u32 10 ("毫秒倍数")) -> ()  [unwired: 1 out]
      }
    }
    frame Enabled {
    }
  }
  n1505 = Obtain Notifier(name (unnamed)=w2, notification data type=w2) -> (notifier out=w1:refnum<notifier>)  [unwired: 2 in, 2 out]
  n1506 = while {
    tunnel: w15 -> [w520]
    tunnel: w14 -> [w519]
    tunnel: [w518] -> w13
    tunnel: [w517] -> w12
    tunnel: w1 -> [w516]
    stop <- w522 stop-if-true
    n1507 = Wait Until Next ms Multiple(millisecond multiple=u32 5 ("毫秒倍数")) -> ()  [unwired: 1 out]
    n1508 = Wait on Notification(notifier=w520, timeout in ms (-1)=20 ("超时毫秒(-1)"), error in (no error)=w519) -> (notifier out=w518:refnum<notifier>, notification=w526:string, error out=w517:errorcluster)  [unwired: 1 in, 1 out]
    n1509 = Equal?(x=w526, y="DInput" ("通知")) -> (x = y?=w521:bool)
    n1510 = case shown="真" w521 {
      tunnel: w516 -> [_ w527]
      frame False {
      }
      frame True {
        n1511 = while {
          tunnel: w527 -> [w528]
          stop <- w529 stop-if-true
          n1512 = stacked-sequence {
            tunnel: [w531 _] -> w529
            tunnel: w528 -> [_ w542]
            frame #0 {
              n1513 = local read "保持输入"() -> (w534:bool)
              n1514 = case shown="假" w534 {
                selector: w534 -> [_ w540]
                tunnel: [w537 w539] -> w533
                frame False {
                  n1515 = local read "同步_A1"() -> (w536:i32)
                  n1516 = Equal?(x=w536, y=5) -> (x = y?=w537:bool)
                }
                frame True {
                  n1517 = Not(x=w540) -> (.not. x?=w539:bool)
                }
              }
              n1518 = local read "关闭？"() -> (w532:bool)
              n1519 = Or(x=w533, y=w532) -> (x .or. y?=w531:bool)
              n1520 = case shown="真" w531 {
                frame False {
                }
                frame True {
                  n1521 = property on="保持输入" class="Bool (严格)"("DisabledEnum"=T1."Enabled" ("禁用")) -> ()  [unwired: 2 in, 2 out]
                }
              }
            }
            frame #1 {
              n1522 = local read "保持输入"() -> (w543:bool)
              n1523 = local read "同步_A1"() -> (w541:i32)
              n1524 = case shown="假" w543 {
                tunnel: w541 -> [w552 _]
                tunnel: [w547 TRUE] -> w544
                frame False {
                  n1525 = local read "同步_A2"() -> (w551:i32)
                  n1526 = Equal?(x=w552, y=w551) -> (x = y?=w549:bool)
                  n1527 = Less?(x=w551, y=5) -> (x < y?=w548:bool)
                  n1528 = And(x=w549, y=w548) -> (x .and. y?=w547:bool)
                }
                frame True {
                }
              }
              n1529 = local read "数组_选择?"() -> (w546:bool[][])
              n1530 = local read "数组_输入值"() -> (w545:enum16{"0", "1"}[][])
              n1531 = case shown="真" w544 {
                tunnel: w546 -> [_ w557]
                tunnel: w541 -> [_ w554]
                tunnel: w545 -> [_ w559]
                tunnel: w542 -> [_ w555]
                frame False {
                }
                frame True {
                  n1532 = Index Array(array=w557, index (row)=w554) -> (element=w556:bool[])  [unwired: 1 in]
                  n1533 = Index Array(array=w559, index (row)=w554) -> (element=w558:enum16{"0", "1"}[])  [unwired: 1 in]
                  n1534 = Or Array Elements(Boolean array=w556) -> (logical OR=w560:bool)
                  n1535 = case shown="真" w560 {
                    tunnel: w558 -> [_ w569]
                    tunnel: w554 -> [_ w570]
                    tunnel: w555 -> [_ w567]
                    frame False {
                      n1536 = local read "保持输入"() -> (w561:bool)
                      n1537 = case shown="假" w561 {
                        frame False {
                          n1538 = local read "同步_A1"() -> (w564:i32)
                          n1539 = local read "同步_A2"() -> (w562:i32)
                          n1540 = Increment(x=w562) -> (x+1=w563:i32)
                          n1541 = Increment(x=w564) -> (x+1=w565:i32)
                          n1542 = local write "同步_A2"(w563) -> ()
                          n1543 = local write "同步_A1"(w565) -> ()
                        }
                        frame True {
                        }
                      }
                    }
                    frame True {
                      n1544 = local read "CAN端口"() -> (w571:u16)
                      n1545 = Increment(x=w570) -> (x+1=w568:i32)
                      n1546 = call "16路数字量输入.vi"("第几组数据"=w568, "CAN端口"=w571) -> ("成功?"=w566:bool)  [unwired: 9 in]
                      n1547 = case shown="真" w566 {
                        tunnel: w569 -> [_ w578]
                        tunnel: w567 -> [_ w577]
                        frame False {
                          n1548 = local read "保持输入"() -> (w572:bool)
                          n1549 = case shown="假" w572 {
                            frame False {
                              n1550 = local read "同步_A1"() -> (w575:i32)
                              n1551 = local read "同步_A2"() -> (w573:i32)
                              n1552 = Increment(x=w575) -> (x+1=w576:i32)
                              n1553 = Increment(x=w573) -> (x+1=w574:i32)
                              n1554 = local write "同步_A2"(w574) -> ()
                              n1555 = local write "同步_A1"(w576) -> ()
                            }
                            frame True {
                            }
                          }
                        }
                        frame True {
                          n1556 = stacked-sequence {
                            tunnel: w578 -> [w583 _ _ _ _ _]
                            tunnel: w577 -> [_ w589 w608 _ _ _]
                            frame #0 {
                              n1557 = for {
                                tunnel: w583 -> [w586] mode=indexing
                                tunnel: [w585] -> w584 mode=indexing
                                n1558 = case shown="\"1\"" w586 {
                                tunnel: [FALSE TRUE] -> w585
                                frame "0", Default {
                                }
                                frame "1" {
                                }
                                }
                              }
                              n1559 = Boolean Array To Number ("布尔数组至数值转换")(Boolean array=w584) -> (number=w582:u16)
                              n1560 = Split Number(x=w582) -> (hi(x)=w579:u8, lo(x)=w580:u8)
                              n1561 = Build Array(w580, w579) -> (w581:u8[])
                              n1562 = call "DO"("dataIn(U8Array)"=w581) -> ()  [unwired: 2 in, 17 out]
                            }
                            frame #1 {
                              # "修改I/O标志"
                              n1563 = local read "同步_A1"() -> (w594:i32)
                              n1564 = Equal?(x=w594, y=4) -> (x = y?=w592:bool)
                              n1565 = Equal?(x=w594, y=5) -> (x = y?=w591:bool)
                              n1566 = Or(x=w592, y=w591) -> (x .or. y?=w590:bool)
                              n1567 = case shown="真" w590 {
                                tunnel: w589 -> [_ w596]
                                frame False {
                                }
                                frame True {
                                n1568 = stacked-sequence {
                                tunnel: w596 -> [w597 _ _ _]
                                frame #0 {
                                n1569 = Send Notification(notification="IOCheck" ("通知"), notifier=w597) -> ()  [unwired: 1 in, 2 out]
                                }
                                frame #1 {
                                n1570 = Wait Until Next ms Multiple(millisecond multiple=u32 10 ("毫秒倍数")) -> ()  [unwired: 1 out]
                                }
                                frame #2 {
                                n1571 = Build Array(u16 54, u16 0, u16 0) -> (w600:u16[])
                                n1572 = call "UDP发送.vi"("发送数据"=w600, "数据区字长"=u16 3, "报文类型"=u16 1285, "发送方标识"=u16 5397) -> ()  [unwired: 6 in, 1 out]
                                }
                                frame #3 {
                                n1573 = Wait (ms)(milliseconds to wait=u32 500 ("毫秒倍数")) -> ()  [unwired: 1 out]
                                }
                                }
                                }
                              }
                            }
                            frame #2 {
                              n1574 = Send Notification(notification="DICheck" ("通知"), notifier=w608) -> ()  [unwired: 1 in, 2 out]
                            }
                            frame #3 {
                              n1575 = Wait (ms)(milliseconds to wait=u32 5 ("等待时间（毫秒）")) -> ()  [unwired: 1 out]
                            }
                            frame #4 {
                              # "双向"
                              # "以太网请求反馈数据"
                              n1576 = Build Array(u16 1024, u16 1025, u16 54) -> (w617:u16[])
                              n1577 = call "UDP发送.vi"("发送数据"=w617, "数据区字长"=u16 3, "报文类型"=u16 2056, "发送方标识"=u16 5397) -> ()  [unwired: 6 in, 1 out]
                            }
                            frame #5 {
                              n1578 = local read "保持输入"() -> (w618:bool)
                              n1579 = case shown="假" w618 {
                                frame False {
                                n1580 = local read "同步_A1"() -> (w619:i32)
                                n1581 = Increment(x=w619) -> (x+1=w620:i32)
                                n1582 = local write "同步_A1"(w620) -> ()
                                }
                                frame True {
                                }
                              }
                            }
                          }
                        }
                      }
                    }
                  }
                }
              }
            }
          }
          n1583 = Wait Until Next ms Multiple(millisecond multiple=u32 5 ("毫秒倍数")) -> ()  [unwired: 1 out]
        }
      }
    }
    n1584 = local read "关闭？"() -> (w522:bool)
  }
  n1585 = Release Notifier(notifier=w13, error in (no error)=w12) -> ()  [unwired: 1 in, 3 out]
  n1586 = disable-structure shown="禁用" {
    frame Disabled {
      n1587 = for {
        N: 40 -> [_]
        i -> [w626]
        n1588 = Wait Until Next ms Multiple(millisecond multiple=u32 10 ("毫秒倍数")) -> ()  [unwired: 1 out]
        n1589 = Bundle(w626, "y"=-1) -> (w625:cluster{i32, "y":i32})  [unwired: 1 in]
        n1590 = property on="D_IN_1" class="Tbl (严格)"("Active Cell"=w625) -> (error out=w624:errorcluster)  [unwired: 2 in, 1 out]
        n1591 = property on="D_IN_1" class="Tbl (严格)"(error in=w624, "Cell BG Color"=u32 12369084) -> ()  [unwired: 1 in, 2 out]
      }
    }
    frame Enabled {
    }
  }
  n1592 = Obtain Notifier(name (unnamed)=w10, notification data type=w10) -> (notifier out=w7:refnum<notifier>, error out=w6:errorcluster)  [unwired: 2 in, 1 out]
  n1593 = while {
    tunnel: [w632] -> w9
    tunnel: [w631] -> w8
    tunnel: w7 -> [w630]
    tunnel: w6 -> [w629]
    stop <- w636 stop-if-true
    n1594 = Wait Until Next ms Multiple(millisecond multiple=u32 5 ("毫秒倍数")) -> ()  [unwired: 1 out]
    n1595 = Wait on Notification(notifier=w630, timeout in ms (-1)=20 ("超时毫秒(-1)"), error in (no error)=w629) -> (notifier out=w632:refnum<notifier>, notification=w628:string, error out=w631:errorcluster)  [unwired: 1 in, 1 out]
    n1596 = Equal?(x=w628, y="DICheck" ("通知")) -> (x = y?=w634:bool)
    n1597 = case shown="真" w634 {
      frame False {
      }
      frame True {
        n1598 = stacked-sequence {
          frame #0 {
            w642 = u16 6
            w650 = u16 5397
            # "错误报文类型"
            # "待定"
            n1599 = local read "保持输入"() -> (w643:bool)
            n1600 = Build Array(w650, u16 34952, u16 0 ("元素")) -> (w647:u16[])
            n1601 = case shown="假" w643 {
              tunnel: [w653 w654] -> w644
              frame False {
                n1602 = local read "同步_A2"() -> (w653:i32)
              }
              frame True {
                n1603 = local read "同步_A1"() -> (w654:i32)
              }
            }
            n1604 = Build Array(w650, u16 2056, w642) -> (w651:u16[])
            n1605 = Add(x=w642, y=u16 4) -> (x+y=w640:u16)
            n1606 = call "UDP接收.vi"("匹配帧信息_异常"=w647, "长度"=w640, "匹配帧信息_正常"=w651) -> ("异常_找到?"=w646:bool, "接收超时?"=w645:bool, "接收的一帧数据"=w639:u16[], "正常_找到?"=w638:bool)  [unwired: 5 in]
            n1607 = case shown="真" w646 {
              frame False {
              }
              frame True {
                n1608 = call "对话框"("Message"="数字量输入返回数值异常") -> ()  [unwired: 9 in, 2 out]
              }
            }
            n1609 = case shown="真" w645 {
              frame False {
              }
              frame True {
                n1610 = call "对话框2"("Message"="以太网接收数据超时失败") -> ()  [unwired: 9 in, 2 out]
              }
            }
            n1611 = case shown="真" w638 {
              tunnel: w639 -> [_ w658]
              tunnel: w642 -> [_ w673]
              tunnel: w644 -> [_ w657]
              frame False {
              }
              frame True {
                n1612 = To Long Integer(number=w673) -> (32bit integer=w662:i32)
                n1613 = Array Subset(array=w658, index=3 ("索引"), length=w662) -> (w659:u16[])
                n1614 = local read "数组_输入值"() -> (w664:enum16{"0", "1"}[][])
                n1615 = local read "数组_选择?"() -> (w663:bool[][])
                n1616 = call "更改输入顺序.vi"("输入数据"=w659) -> ("更改顺序后数据"=w661:u16[])  [unwired: 10 in]
                n1617 = Index Array(array=w663, index (row)=w657) -> (element=w667:bool[])  [unwired: 1 in]
                n1618 = Index Array(array=w664, index (row)=w657) -> (element=w666:enum16{"0", "1"}[])  [unwired: 1 in]
                n1619 = Index Array(array=w661, index=w657) -> (element=w660:u16)
                n1620 = Number To Boolean Array(number=w660) -> (Boolean array=w671:bool[])
                n1621 = call "16路数字量输入判断.vi"("反馈值"=w671, "输入值"=w666, "是否选择"=w667) -> ("合格"=w668:bool, "结果"=w670:cluster{u32, u32}[][], "反馈值字符串"=w669:string[])  [unwired: 6 in]
                n1622 = case shown="4" w657 {
                  tunnel: w670 -> [w675 w732 w769 w806 w843]
                  tunnel: w669 -> [w677 w713 w750 w786 w823]
                  frame 0, Default {
                    n1623 = local read "D_IN_1"() -> (w679:string[][])
                    n1624 = Replace Array Subset(array=w679, new element=w677, index (col)=2 ("禁用的索引 (列)")) -> (w676:string[][])  [unwired: 1 in]
                    n1625 = Index Array(array=w675, index (row) #1=0 ("索引"), index (row) #2=1 ("索引"), index (row) #3=2 ("索引"), index (row) #4=3 ("索引"), index (row) #5=4 ("索引"), index (row) #6=5 ("索引"), index (row) #7=6 ("索引"), index (row) #8=7 ("索引"), index (row) #9=8 ("索引"), index (row) #10=9 ("索引"), index (row) #11=10 ("索引"), index (row) #12=11 ("索引"), index (row) #13=12 ("索引"), index (row) #14=13 ("索引"), index (row) #15=14 ("索引"), index (row) #16=15 ("索引")) -> (element #1=w695:cluster{u32, u32}[], element #2=w694:cluster{u32, u32}[], element #3=w693:cluster{u32, u32}[], element #4=w692:cluster{u32, u32}[], element #5=w691:cluster{u32, u32}[], element #6=w680:cluster{u32, u32}[], element #7=w681:cluster{u32, u32}[], element #8=w682:cluster{u32, u32}[], element #9=w683:cluster{u32, u32}[], element #10=w684:cluster{u32, u32}[], element #11=w685:cluster{u32, u32}[], element #12=w686:cluster{u32, u32}[], element #13=w687:cluster{u32, u32}[], element #14=w688:cluster{u32, u32}[], element #15=w689:cluster{u32, u32}[], element #16=w690:cluster{u32, u32}[])  [unwired: 16 in]
                    n1626 = local write "D_IN_1"(w676) -> ()
                    n1627 = property on="light_1" class="Bool (严格)"("Colors [4]"=w695) -> ()  [unwired: 2 in, 2 out]
                    n1628 = property on="light_2" class="Bool (严格)"("Colors [4]"=w694) -> ()  [unwired: 2 in, 2 out]
                    n1629 = property on="light_3" class="Bool (严格)"("Colors [4]"=w693) -> ()  [unwired: 2 in, 2 out]
                    n1630 = property on="light_4" class="Bool (严格)"("Colors [4]"=w692) -> ()  [unwired: 2 in, 2 out]
                    n1631 = property on="light_5" class="Bool (严格)"("Colors [4]"=w691) -> ()  [unwired: 2 in, 2 out]
                    n1632 = property on="light_6" class="Bool (严格)"("Colors [4]"=w680) -> ()  [unwired: 2 in, 2 out]
                    n1633 = property on="light_7" class="Bool (严格)"("Colors [4]"=w681) -> ()  [unwired: 2 in, 2 out]
                    n1634 = property on="light_8" class="Bool (严格)"("Colors [4]"=w682) -> ()  [unwired: 2 in, 2 out]
                    n1635 = property on="light_9" class="Bool (严格)"("Colors [4]"=w683) -> ()  [unwired: 2 in, 2 out]
                    n1636 = property on="light_10" class="Bool (严格)"("Colors [4]"=w684) -> ()  [unwired: 2 in, 2 out]
                    n1637 = property on="light_11" class="Bool (严格)"("Colors [4]"=w685) -> ()  [unwired: 2 in, 2 out]
                    n1638 = property on="light_12" class="Bool (严格)"("Colors [4]"=w686) -> ()  [unwired: 2 in, 2 out]
                    n1639 = property on="light_13" class="Bool (严格)"("Colors [4]"=w687) -> ()  [unwired: 2 in, 2 out]
                    n1640 = property on="light_14" class="Bool (严格)"("Colors [4]"=w688) -> ()  [unwired: 2 in, 2 out]
                    n1641 = property on="light_15" class="Bool (严格)"("Colors [4]"=w689) -> ()  [unwired: 2 in, 2 out]
                    n1642 = property on="light_16" class="Bool (严格)"("Colors [4]"=w690) -> ()  [unwired: 2 in, 2 out]
                  }
                  frame 2 {
                    n1643 = local read "D_IN_3"() -> (w714:string[][])
                    n1644 = Replace Array Subset(array=w714, new element=w713, index (col)=2 ("索引 (列)")) -> (w712:string[][])  [unwired: 1 in]
                    n1645 = Index Array(array=w732, index (row) #1=0 ("索引"), index (row) #2=1 ("索引"), index (row) #3=2 ("索引"), index (row) #4=3 ("索引"), index (row) #5=4 ("索引"), index (row) #6=5 ("索引"), index (row) #7=6 ("索引"), index (row) #8=7 ("索引"), index (row) #9=8 ("索引"), index (row) #10=9 ("索引"), index (row) #11=10 ("索引"), index (row) #12=11 ("索引"), index (row) #13=12 ("索引"), index (row) #14=13 ("索引"), index (row) #15=14 ("索引"), index (row) #16=15 ("索引")) -> (element #1=w731:cluster{u32, u32}[], element #2=w730:cluster{u32, u32}[], element #3=w729:cluster{u32, u32}[], element #4=w728:cluster{u32, u32}[], element #5=w727:cluster{u32, u32}[], element #6=w726:cluster{u32, u32}[], element #7=w725:cluster{u32, u32}[], element #8=w724:cluster{u32, u32}[], element #9=w723:cluster{u32, u32}[], element #10=w722:cluster{u32, u32}[], element #11=w721:cluster{u32, u32}[], element #12=w720:cluster{u32, u32}[], element #13=w719:cluster{u32, u32}[], element #14=w718:cluster{u32, u32}[], element #15=w717:cluster{u32, u32}[], element #16=w716:cluster{u32, u32}[])  [unwired: 16 in]
                    n1646 = local write "D_IN_3"(w712) -> ()
                    n1647 = property on="light_33" class="Bool (严格)"("Colors [4]"=w731) -> ()  [unwired: 2 in, 2 out]
                    n1648 = property on="light_34" class="Bool (严格)"("Colors [4]"=w730) -> ()  [unwired: 2 in, 2 out]
                    n1649 = property on="light_35" class="Bool (严格)"("Colors [4]"=w729) -> ()  [unwired: 2 in, 2 out]
                    n1650 = property on="light_36" class="Bool (严格)"("Colors [4]"=w728) -> ()  [unwired: 2 in, 2 out]
                    n1651 = property on="light_37" class="Bool (严格)"("Colors [4]"=w727) -> ()  [unwired: 2 in, 2 out]
                    n1652 = property on="light_38" class="Bool (严格)"("Colors [4]"=w726) -> ()  [unwired: 2 in, 2 out]
                    n1653 = property on="light_39" class="Bool (严格)"("Colors [4]"=w725) -> ()  [unwired: 2 in, 2 out]
                    n1654 = property on="light_40" class="Bool (严格)"("Colors [4]"=w724) -> ()  [unwired: 2 in, 2 out]
                    n1655 = property on="light_41" class="Bool (严格)"("Colors [4]"=w723) -> ()  [unwired: 2 in, 2 out]
                    n1656 = property on="light_42" class="Bool (严格)"("Colors [4]"=w722) -> ()  [unwired: 2 in, 2 out]
                    n1657 = property on="light_43" class="Bool (严格)"("Colors [4]"=w721) -> ()  [unwired: 2 in, 2 out]
                    n1658 = property on="light_44" class="Bool (严格)"("Colors [4]"=w720) -> ()  [unwired: 2 in, 2 out]
                    n1659 = property on="light_45" class="Bool (严格)"("Colors [4]"=w719) -> ()  [unwired: 2 in, 2 out]
                    n1660 = property on="light_46" class="Bool (严格)"("Colors [4]"=w718) -> ()  [unwired: 2 in, 2 out]
                    n1661 = property on="light_47" class="Bool (严格)"("Colors [4]"=w717) -> ()  [unwired: 2 in, 2 out]
                    n1662 = property on="light_48" class="Bool (严格)"("Colors [4]"=w716) -> ()  [unwired: 2 in, 2 out]
                  }
                  frame 3 {
                    n1663 = local read "D_IN_4"() -> (w751:string[][])
                    n1664 = Replace Array Subset(array=w751, new element=w750, index (col)=2 ("索引 (列)")) -> (w749:string[][])  [unwired: 1 in]
                    n1665 = Index Array(array=w769, index (row) #1=0 ("索引"), index (row) #2=1 ("索引"), index (row) #3=2 ("索引"), index (row) #4=3 ("索引"), index (row) #5=4 ("索引"), index (row) #6=5 ("索引"), index (row) #7=6 ("索引"), index (row) #8=7 ("索引"), index (row) #9=8 ("索引"), index (row) #10=9 ("索引"), index (row) #11=10 ("索引"), index (row) #12=11 ("索引"), index (row) #13=12 ("索引"), index (row) #14=13 ("索引"), index (row) #15=14 ("索引"), index (row) #16=15 ("索引")) -> (element #1=w768:cluster{u32, u32}[], element #2=w767:cluster{u32, u32}[], element #3=w766:cluster{u32, u32}[], element #4=w765:cluster{u32, u32}[], element #5=w764:cluster{u32, u32}[], element #6=w763:cluster{u32, u32}[], element #7=w762:cluster{u32, u32}[], element #8=w761:cluster{u32, u32}[], element #9=w760:cluster{u32, u32}[], element #10=w759:cluster{u32, u32}[], element #11=w758:cluster{u32, u32}[], element #12=w757:cluster{u32, u32}[], element #13=w756:cluster{u32, u32}[], element #14=w755:cluster{u32, u32}[], element #15=w754:cluster{u32, u32}[], element #16=w753:cluster{u32, u32}[])  [unwired: 16 in]
                    n1666 = local write "D_IN_4"(w749) -> ()
                    n1667 = property on="light_49" class="Bool (严格)"("Colors [4]"=w768) -> ()  [unwired: 2 in, 2 out]
                    n1668 = property on="light_50" class="Bool (严格)"("Colors [4]"=w767) -> ()  [unwired: 2 in, 2 out]
                    n1669 = property on="light_51" class="Bool (严格)"("Colors [4]"=w766) -> ()  [unwired: 2 in, 2 out]
                    n1670 = property on="light_52" class="Bool (严格)"("Colors [4]"=w765) -> ()  [unwired: 2 in, 2 out]
                    n1671 = property on="light_53" class="Bool (严格)"("Colors [4]"=w764) -> ()  [unwired: 2 in, 2 out]
                    n1672 = property on="light_54" class="Bool (严格)"("Colors [4]"=w763) -> ()  [unwired: 2 in, 2 out]
                    n1673 = property on="light_55" class="Bool (严格)"("Colors [4]"=w762) -> ()  [unwired: 2 in, 2 out]
                    n1674 = property on="light_56" class="Bool (严格)"("Colors [4]"=w761) -> ()  [unwired: 2 in, 2 out]
                    n1675 = property on="light_57" class="Bool (严格)"("Colors [4]"=w760) -> ()  [unwired: 2 in, 2 out]
                    n1676 = property on="light_58" class="Bool (严格)"("Colors [4]"=w759) -> ()  [unwired: 2 in, 2 out]
                    n1677 = property on="light_59" class="Bool (严格)"("Colors [4]"=w758) -> ()  [unwired: 2 in, 2 out]
                    n1678 = property on="light_60" class="Bool (严格)"("Colors [4]"=w757) -> ()  [unwired: 2 in, 2 out]
                    n1679 = property on="light_61" class="Bool (严格)"("Colors [4]"=w756) -> ()  [unwired: 2 in, 2 out]
                    n1680 = property on="light_62" class="Bool (严格)"("Colors [4]"=w755) -> ()  [unwired: 2 in, 2 out]
                    n1681 = property on="light_63" class="Bool (严格)"("Colors [4]"=w754) -> ()  [unwired: 2 in, 2 out]
                    n1682 = property on="light_64" class="Bool (严格)"("Colors [4]"=w753) -> ()  [unwired: 2 in, 2 out]
                  }
                  frame 4 {
                    n1683 = local read "D_IN_5"() -> (w788:string[][])
                    n1684 = Replace Array Subset(array=w788, new element=w786, index (col)=2 ("索引 (列)")) -> (w787:string[][])  [unwired: 1 in]
                    n1685 = Index Array(array=w806, index (row) #1=0 ("索引"), index (row) #2=1 ("索引"), index (row) #3=2 ("索引"), index (row) #4=3 ("索引"), index (row) #5=4 ("索引"), index (row) #6=5 ("索引"), index (row) #7=6 ("索引"), index (row) #8=7 ("索引"), index (row) #9=8 ("索引"), index (row) #10=9 ("索引"), index (row) #11=10 ("索引"), index (row) #12=11 ("索引"), index (row) #13=12 ("索引"), index (row) #14=13 ("索引"), index (row) #15=14 ("索引"), index (row) #16=15 ("索引")) -> (element #1=w805:cluster{u32, u32}[], element #2=w804:cluster{u32, u32}[], element #3=w803:cluster{u32, u32}[], element #4=w802:cluster{u32, u32}[], element #5=w801:cluster{u32, u32}[], element #6=w800:cluster{u32, u32}[], element #7=w799:cluster{u32, u32}[], element #8=w798:cluster{u32, u32}[], element #9=w797:cluster{u32, u32}[], element #10=w796:cluster{u32, u32}[], element #11=w795:cluster{u32, u32}[], element #12=w794:cluster{u32, u32}[], element #13=w793:cluster{u32, u32}[], element #14=w792:cluster{u32, u32}[], element #15=w791:cluster{u32, u32}[], element #16=w790:cluster{u32, u32}[])  [unwired: 16 in]
                    n1686 = local write "D_IN_5"(w787) -> ()
                    n1687 = property on="light_65" class="Bool (严格)"("Colors [4]"=w805) -> ()  [unwired: 2 in, 2 out]
                    n1688 = property on="light_66" class="Bool (严格)"("Colors [4]"=w804) -> ()  [unwired: 2 in, 2 out]
                    n1689 = property on="light_67" class="Bool (严格)"("Colors [4]"=w803) -> ()  [unwired: 2 in, 2 out]
                    n1690 = property on="light_68" class="Bool (严格)"("Colors [4]"=w802) -> ()  [unwired: 2 in, 2 out]
                    n1691 = property on="light_69" class="Bool (严格)"("Colors [4]"=w801) -> ()  [unwired: 2 in, 2 out]
                    n1692 = property on="light_70" class="Bool (严格)"("Colors [4]"=w800) -> ()  [unwired: 2 in, 2 out]
                    n1693 = property on="light_71" class="Bool (严格)"("Colors [4]"=w799) -> ()  [unwired: 2 in, 2 out]
                    n1694 = property on="light_72" class="Bool (严格)"("Colors [4]"=w798) -> ()  [unwired: 2 in, 2 out]
                    n1695 = property on="light_73" class="Bool (严格)"("Colors [4]"=w797) -> ()  [unwired: 2 in, 2 out]
                    n1696 = property on="light_74" class="Bool (严格)"("Colors [4]"=w796) -> ()  [unwired: 2 in, 2 out]
                    n1697 = property on="light_75" class="Bool (严格)"("Colors [4]"=w795) -> ()  [unwired: 2 in, 2 out]
                    n1698 = property on="light_76" class="Bool (严格)"("Colors [4]"=w794) -> ()  [unwired: 2 in, 2 out]
                    n1699 = property on="light_77" class="Bool (严格)"("Colors [4]"=w793) -> ()  [unwired: 2 in, 2 out]
                    n1700 = property on="light_78" class="Bool (严格)"("Colors [4]"=w792) -> ()  [unwired: 2 in, 2 out]
                    n1701 = property on="light_79" class="Bool (严格)"("Colors [4]"=w791) -> ()  [unwired: 2 in, 2 out]
                    n1702 = property on="light_80" class="Bool (严格)"("Colors [4]"=w790) -> ()  [unwired: 2 in, 2 out]
                  }
                  frame 1 {
                    n1703 = local read "D_IN_2"() -> (w825:string[][])
                    n1704 = Replace Array Subset(array=w825, new element=w823, index (col)=2 ("索引 (列)")) -> (w824:string[][])  [unwired: 1 in]
                    n1705 = Index Array(array=w843, index (row) #1=0 ("索引"), index (row) #2=1 ("索引"), index (row) #3=2 ("索引"), index (row) #4=3 ("索引"), index (row) #5=4 ("索引"), index (row) #6=5 ("索引"), index (row) #7=6 ("索引"), index (row) #8=7 ("索引"), index (row) #9=8 ("索引"), index (row) #10=9 ("索引"), index (row) #11=10 ("索引"), index (row) #12=11 ("索引"), index (row) #13=12 ("索引"), index (row) #14=13 ("索引"), index (row) #15=14 ("索引"), index (row) #16=15 ("索引")) -> (element #1=w842:cluster{u32, u32}[], element #2=w841:cluster{u32, u32}[], element #3=w840:cluster{u32, u32}[], element #4=w839:cluster{u32, u32}[], element #5=w838:cluster{u32, u32}[], element #6=w837:cluster{u32, u32}[], element #7=w836:cluster{u32, u32}[], element #8=w835:cluster{u32, u32}[], element #9=w834:cluster{u32, u32}[], element #10=w833:cluster{u32, u32}[], element #11=w832:cluster{u32, u32}[], element #12=w831:cluster{u32, u32}[], element #13=w830:cluster{u32, u32}[], element #14=w829:cluster{u32, u32}[], element #15=w828:cluster{u32, u32}[], element #16=w827:cluster{u32, u32}[])  [unwired: 16 in]
                    n1706 = local write "D_IN_2"(w824) -> ()
                    n1707 = property on="light_17" class="Bool (严格)"("Colors [4]"=w842) -> ()  [unwired: 2 in, 2 out]
                    n1708 = property on="light_18" class="Bool (严格)"("Colors [4]"=w841) -> ()  [unwired: 2 in, 2 out]
                    n1709 = property on="light_19" class="Bool (严格)"("Colors [4]"=w840) -> ()  [unwired: 2 in, 2 out]
                    n1710 = property on="light_20" class="Bool (严格)"("Colors [4]"=w839) -> ()  [unwired: 2 in, 2 out]
                    n1711 = property on="light_21" class="Bool (严格)"("Colors [4]"=w838) -> ()  [unwired: 2 in, 2 out]
                    n1712 = property on="light_22" class="Bool (严格)"("Colors [4]"=w837) -> ()  [unwired: 2 in, 2 out]
                    n1713 = property on="light_23" class="Bool (严格)"("Colors [4]"=w836) -> ()  [unwired: 2 in, 2 out]
                    n1714 = property on="light_24" class="Bool (严格)"("Colors [4]"=w835) -> ()  [unwired: 2 in, 2 out]
                    n1715 = property on="light_25" class="Bool (严格)"("Colors [4]"=w834) -> ()  [unwired: 2 in, 2 out]
                    n1716 = property on="light_26" class="Bool (严格)"("Colors [4]"=w833) -> ()  [unwired: 2 in, 2 out]
                    n1717 = property on="light_27" class="Bool (严格)"("Colors [4]"=w832) -> ()  [unwired: 2 in, 2 out]
                    n1718 = property on="light_28" class="Bool (严格)"("Colors [4]"=w831) -> ()  [unwired: 2 in, 2 out]
                    n1719 = property on="light_29" class="Bool (严格)"("Colors [4]"=w830) -> ()  [unwired: 2 in, 2 out]
                    n1720 = property on="light_30" class="Bool (严格)"("Colors [4]"=w829) -> ()  [unwired: 2 in, 2 out]
                    n1721 = property on="light_31" class="Bool (严格)"("Colors [4]"=w828) -> ()  [unwired: 2 in, 2 out]
                    n1722 = property on="light_32" class="Bool (严格)"("Colors [4]"=w827) -> ()  [unwired: 2 in, 2 out]
                  }
                }
                n1723 = local read "测试结论"() -> (w665:string)
                n1724 = case shown="真" w668 {
                  tunnel: [w865 w871] -> w672
                  tunnel: w665 -> [w866 w872]
                  tunnel: w657 -> [w861 w869]
                  frame False {
                    n1725 = Increment(x=w861) -> (x+1=w860:i32)
                    n1726 = Format Into String(format string="被测板卡第%d路数字量输入测试故障，\n具体见上面试验结论！", w860) -> (resulting string=w863:string)  [unwired: 2 in, 1 out]
                    n1727 = Concatenate Strings(w866, w863, "\r") -> (w865:string)
                  }
                  frame True {
                    n1728 = Format Into String(format string="被测板卡第%d路数字量输入正常！", w869) -> (resulting string=w868:string)  [unwired: 2 in, 1 out]
                    n1729 = Concatenate Strings(w872, w868, "\r") -> (w871:string)
                  }
                }
                n1730 = local write "测试结论"(w672) -> ()
              }
            }
          }
          frame #1 {
            n1731 = local read "保持输入"() -> (w873:bool)
            n1732 = case shown="假" w873 {
              frame False {
                n1733 = local read "同步_A2"() -> (w875:i32)
                n1734 = Increment(x=w875) -> (x+1=w874:i32)
                n1735 = local write "同步_A2"(w874) -> ()
              }
              frame True {
              }
            }
          }
        }
      }
    }
    n1736 = local read "关闭？"() -> (w636:bool)
  }
  n1737 = Release Notifier(notifier=w9, error in (no error)=w8) -> ()  [unwired: 1 in, 3 out]
